vi "UHR-Fleezers Control (fpga) - Leonardo 04-2018 V4b_AlexFCS.vi"() -> ()   [LabVIEW 2013]
doc: "UHR-Fleezers Instrument Control Code (fpga)"
uses:
  <vilib>/Platform/TimedLoop/XDataNode/timing_clust.ctl
  <vilib>/Platform/TimedLoop/XDataNode/nitl_modes.ctl
  <vilib>/Platform/TimedLoop/XDataNode/wakeup.ctl
  <vilib>/rvi/eio/common/nirviEmuTemplateMethod_errors.vi
  <vilib>/rvi/Emulation/niFpgaSctlEmulationGetInTimedLoop.vi
  <vilib>/rvi/Emulation/niFpgaEmulationReportErrorSimple.vi
  <vilib>/rvi/Emulation/niFpgaGetClockAttributes.vi
  <vilib>/rvi/Emulation/niFpgaCriticalErrorInLSC.vi
  <vilib>/rvi/FIFO/Fifo_Resource/nirvififoEmulationReadFpgaImpl.vi
  <vilib>/rvi/DataTransferAndStorage/Container/Common/niFpgaContainerGetUniqueNameForEmu.vi
  <vilib>/rvi/DataTransferAndStorage/Container/Common/niFpgaContainerExecOnDevCompGetState.vi
  <vilib>/rvi/interface/RandomDataEmulation/nirviRandomDataFPGAFIFO.vi
  <vilib>/rvi/interface/RandomDataEmulation/niFpgaRandomDataHandleErrors.vi
  <vilib>/rvi/eio/common/nirviEmuReportErrorAndStop.vi
  <vilib>/rvi/FIFO/Fifo_Resource/nirvififoEmulationGetNumberOfElementsToReadFpgaImpl.vi
  <vilib>/rvi/FIFO/Fifo_Resource/nirvififoEmulationClearFpgaImpl.vi
  <vilib>/rvi/Emulation/niFpgaProcessEmulError.vi
  <vilib>/rvi/FIFO/Fifo_Resource/nirvififoEmulationWriteFpgaImpl.vi
  <vilib>/Platform/TimedLoop/XDataNode/XDataNode.xnode
  <vilib>/eio/EIOMethodNode/EIOMethodNode.xnode
  <vilib>/eio/EIONode/EIONode.xnode
  <vilib>/rvi/DataTransferAndStorage/Container/XNode/niFpgaContainer.xnode
  <vilib>/rvi/FIFO/Fifo_Resource/nirvififoEmulationRead.vi
  <vilib>/rvi/FIFO/Fifo_Resource/niFpgaFifoEmulationRefIn.vi
  <vilib>/rvi/FIFO/Fifo_Resource/nirvififoEmulationGetNumberOfElementsToRead.vi
  <vilib>/rvi/interface/RandomDataEmulation/nirviRandomDataFpgaReadWriteTemplate.vi
  <vilib>/rvi/FIFO/Fifo_Resource/nirvififoEmulationWrite.vi
  <vilib>/addons/control/pid/fpga.llb/XNode/niFpgaPID.xnode
  <vilib>/Platform/TimedLoop/XDataNode/XDNodeRunTimeDep.lvlib
  <vilib>/rvi/Memory/Memory_Emulation/niFpgaMemoryEmulationRefIn.vi
panel:
  in  "Tab Control 2":T1(tab)
  out "BD1 amplitude 1 out":u16
  out "BD1 amplitude 2 out":u16
  in  "FB output range":cluster{"output low":i16, "output high":i16}={"output low"=0, "output high"=3000}
  in  "FB Gains":T2={"proportional gain (Kc)"=10, "integral gain (Kc*Ts/Ti)"=5, "derivative gain (Kc*Td/Ts)"=0}
  in  "RF synth green feedback max":i16=4000
  in  "RD":bool=TRUE
  in  "Swap F1 and F2":bool
  in  "Scan BD":bool
  in  "Start scan":bool
  in  "OSK Bd 1":bool
  in  "Reset Bd 1":bool
  in  "PMODE":bool=TRUE
  in  "Number Interlace Cycles":u8=2 min=1 max=3
  in  "Interlace Off Parameters":u8=1 min=1 max=3
  in  "Interlace ON/OFF":bool
  out "DIO Relative phase":i16
  in  "Phase count adjustment (DIO)":i16
  in  "+ phase (DIO)":bool
  out "DIO Late Counter":u8
  in  "DIO count 1 (ticks)":u16=400
  in  "DIO count 2 (ticks)":u16=400
  in  "DIO count 3 (ticks)":u16=400
  out "AI2 Y Sum Set 2":i16
  out "AI2 Y Sum Set 1":i16
  in  "FB Setpoint Set 1":i16 min=0 step=1
  in  "FB Reset Set 1":bool
  in  "FB On/Off Set 1":bool
  in  "FB Reset Set 2":bool
  in  "FB On/Off Set 2":bool
  in  "FB Setpoint Set 2":i16 min=0 step=1
  in  "Amp switch delay":u8=5
  in  "RF synth bd controls green":bool
  in  "Phase Trap 2":fxp<+,14,14>
  in  "Phase Trap 1":fxp<+,14,14>
  in  "Phase offset method":u8
  in  "BD 2 Amplitude 1":u16
  in  "BD 1 Amplitude 1":u16
  in  "BD 2 Frequency 1":u64
  in  "BD 1 Frequency 1":u64
  in  "BD 2 Amplitude 2":u16
  in  "BD 1 Amplitude 2":u16
  in  "BD 2 Frequency 2":u64
  in  "BD 1 Frequency 2":u64
  in  "BD 2 Amplitude 3":u16
  in  "BD 1 Amplitude 3":u16
  in  "BD 2 Frequency 3":u64
  in  "BD 1 Frequency 3":u64
  in  "BD 2 Delay (Ticks)":u8 caption="Count(Ticks)"
  in  "Next trap write delay (ticks)":u8 caption="Count(Ticks)"
  out "Random phase generated":fxp<+,14,14>
  in  "RF phase reset before cycles":bool
  in  "Trap 1 osc enable":bool
  in  "N trap osc periods":i16
  in  "Trap osc period (pts)":i16
  in  "Osc traps":bool
  in  "Initiate trap osc":bool
  in  "Ready Write":bool
  in  "Data":i64
  in  "Address 2":u32
  in  "Osc trap cont.":bool
  in  "Trap 2 osc enable":bool
  out "green FB running":bool
  in  "APD 2 AO scale factor":i16=1
  in  "BD 1 Delay (ticks)":u8
  in  "Tab Control":T3(tab)=enum."MCL trap control"
  in  "Set 3":bool
  in  "Set 2":bool=TRUE
  in  "Set 1":bool=TRUE
  in  "Trap Pos to FIFO":bool
  in  "N of AI1 Int Acq Sets":i16=2 min=1 max=3 step=1
  out "AI Late Counter":u8
  in  "ai count":u16=400
  in  "+ phase":bool
  in  "Phase count adjustment":i16
  out "Relative phase":i16
  in  "AI to FIFO":bool
  out "BD1 Frequency Out 1":u64
  out "BD1 Frequency Out 2":u64
  out "Trap Pos FIFO Timeout":u16
  out "Trap AI FIFO Timeout":u16
  in  "Trap FIFO Set Timeout":i32
  in  "Scan freq.  increment":i64
  in  "Scan steps":u64
  in  "Number of scans":u16
  in  "Cycles per step":u64
  in  "Raster setpoint":fxp<+/-,16,1>
  in  "Raster to target force":bool
  out "Actual Scan freq":u64
  in  "Cont. Scan":bool
  out "Scan I":u64
  in  "Abort scan":bool
  out "Scanning":bool
  in  "FB Min frequency":u64
  in  "FB Max Frequency":u64
  in  "Dynamic Force FB (Ronen)":bool
  in  "Trap pos. FB Range":T4={"FB2 output low"=-1.0, "FB2 output high"=0.999969482421875}
  in  "Trap Pos. FB Gains":T5={"proportional gain (Kc)"=0.999969482421875, "integral gain (Kc*Ts/Ti)"=0.999969482421875, "derivative gain (Kc*Td/Ts)"=0.0}
  in  "B factor":fxp<+/-,32,16>
  in  "Negate Diff?":bool
  in  "Diff FB Measurement?":bool
  in  "FB Trig Integrate":u32=1
  out "TTrig?":bool
  in  "TTrig Negate Pos":bool=TRUE
  out "Trap Pos FB Int Signal":fxp<+/-,24,9> format="%.18g"
  out "Trap Pos FB Int-Norm Signal":fxp<+/-,16,1> format="%.16g"
  in  "FPGA TTrig Thresh":i64
  in  "FPGA Trap Trig":bool
  out "Trap Pos FB Action":i64
  in  "Trap Pos. FB Offset Factor":i64
  in  "Trap Pos. FB Mult Factor":i64=2
  in  "Trap Pos. FB Reset":bool
  in  "Trap Pos FB Monitor T1 or T2":bool
  in  "AI1 X Scale":u16
  in  "Trap Pos FB Int Count":u16=100
  in  "Trap Pos FB Negate Action":bool
  out "AI1 X Set 2":fxp<+/-,16,1>
  out "AI1 X Set 1":fxp<+/-,16,1>
  in  "Trap Pos. FB SP":fxp<+/-,16,1>
  in  "Force feedback":bool
  out "TTrig Sig":i64
  out "TTrig Fin Thresh":i64
  in  "1D or 2D Scan?":bool
  in  "Abort scan (MCL)":bool
  in  "MCL Scan Axis":bool
  in  "Cont. Scan (MCL)":bool
  out "Scan I (MCL)":u64
  in  "Number of scans (MCL)":u16
  out "Scanning MCL":bool
  in  "Scan steps (MCL)":u64
  in  "Cycles per step (MCL)":u64
  in  "Scan freq.  increment (MCL)":i16
  in  "Start scan (MCL)":bool
  in  "AO2 (X)":i16
  in  "AO1 (Y)":i16
  out "MCL Late Counter":u8
  in  "MCL count":u32=800
  out "MCL Relative Phase":i16
  in  "Phase count adjustment (MCL)":i16
  in  "+ phase (MCL)":bool
  in  "Lifetime events to read blue":u16=100
  in  "Lifetime read blue fifo":bool
  out "lifetime events in fifo":u16
  out "APD2 int gate":bool
  in  "APD Gate Operating Mode":u8 max=2 step=1
  in  "Invert APD Gate":bool
  in  "APD Gate OFF Count":u16=100
  in  "APD Gate ON Count":u16=300
  out "APD 1 Gate Late Counter":u8
  out "APD 1 Gate Relative Phase":i16
  in  "Phase count adjustment (APD 1 Gate)":i16
  in  "+ phase (APD 1 Gate)":bool
  in  "Phase count adjustment (APD 2 Gate)":i16
  out "APD 2 Gate Late Counter":u8
  out "APD 2 Gate Relative Phase":i16
  in  "+ phase (APD 2 Gate)":bool
  out "APD 3 Counts 0":u32
  out "APD 3 Counts 1":u32
  out "APD 3 Gate Late Counter":u8
  in  "Phase count adjustment (APD 3 Gate)":i16
  out "APD 3 Gate Relative Phase":i16
  in  "+ phase (APD 3 Gate)":bool
  out "APD1 int gate":bool
  out "APD3 int gate":bool
  in  "Lifetime timeout APD1":u16=200
  in  "APD to FIFO":bool
  in  "APD Acq Rate Count":u32=20000000
  out "APD Acq Late Counter":u16
  out "APD Acq Relative Phase":i16
  in  "+ phase (APD Acq)":bool
  in  "Phase Count Adjustment (APD Acq)":i16
  in  "APD 1 AO scale factor":i16=1
  out "APD Acq Late?":bool
  in  "Number of OFF cycles":i16
  in  "Green long-scale interlacing":bool
  in  "D3 2":i16
  in  "I3 2":i16=5
  in  "P3 2":i16=10
  in  "Green FB Setpoint 2":i16=250 min=0 step=1
  in  "Green FB Reset 2":bool
  in  "Green Filter Flipper":bool
  in  "Green interlace OFF count":u16=100
  out "GI Relative phase":i16
  in  "Phase count adjustment (GI)":i16
  in  "+ phase (GI)":bool
  in  "Green interlace ON count":u16=300
  out "GI Late Counter":u8
  in  "Invert GI":bool
  in  "Operating Mode":u8 max=2 step=1
  in  "Current Out":u16=30000
  in  "Green int current ON count adj":u32=150
  in  "Green interlace OFF count 2":u32=900
  in  "Green interlace ON count 2":u32=300
  out "GI Late Counter 2":u16
  in  "Green FB Count":u32=1200
  in  "Phase count adjustment (GI) 2":i16=20
  in  "Green FB Setpoint":i16=250 min=0 step=1
  in  "Invert GI 2":bool
  out "GI Relative phase 2":i16
  in  "+ phase (GI) 2":bool
  in  "Phase count adjustment (Green FB)":i16=10
  out "Green Late Counter":u16
  out "Green FB Relative Phase":i16
  in  "+ phase (Green FB)":bool
  out "Green FB Signals":T6
  out "Green FB Sum":i16
  in  "Green FB Gains":T2={"proportional gain (Kc)"=10, "integral gain (Kc*Ts/Ti)"=5, "derivative gain (Kc*Td/Ts)"=0}
  in  "Green FB On/Off":bool
  in  "Green FB Reset":bool
  out "Green FB Late?":bool
  out "GI Late?":bool
  in  "Operating Mode 2":u8=2 max=2 step=1
  in  "Chassis2/Mod4/AO1":u16
  in  "Number of ON cycles":i16
  in  "+ phase (RI)":bool
  out "RI Relative phase":i16
  out "RI Late Counter":u8
  in  "Red interlace ON count":u16=300
  in  "Red interlace OFF count":u16=100
  in  "Invert RI":bool
  in  "Red Laser Operating Mode":u8 max=2 step=1
  in  "Phase count adjustment (RI)":i16
  in  "Phase count adjustment (BI D)":i16
  in  "Blue Laser Operating Mode (D)":u8 max=2 step=1
  in  "Invert BI (D)":bool
  in  "Blue interlace OFF count (D)":u16=100
  in  "Blue interlace ON count (D)":u16=300
  out "Blue Late Counter (D)":u8
  out "BI Relative phase (D)":i16
  in  "+ phase (BI D)":bool
  in  "Lifetime to FIFO":bool
  out "lifetime (ticks)":u16
  # "Raster Scan AOD"
  # "1 (X)"
  # "2 (Y)"
  # "IR Intensity Feedback (RF BD 1)"
  # "FB Gains Set 1"
  # "FB output range 1"
  # "IR Intensity Feedback (RF BD 2) -\nonly when using BD 2 for green laser AOM (not trap Y)"
  # "Keep below 4096 (12 bits) to stay within range of RF board. Going over doesn't saturate, it truncates higher bits."
  # "RF phase offset control"
  # "Methods are:\n0 - Default, do nothing at all (no phase offset writes)\n1 - Manual phase adjustment\n2 - Cycle the phase adjustment using the input phase numbers as increment values for each cycle"
  # "False is usual, True is external loop method"
  # "Parameters if using the external RF switching loop"
  # "Parameters if using the usual internal RF switching method"
  # "FB Triggering Excitation Laser"
  # "Trap Pos. FB Gains"
  # "Trap Pos. FB Range"
  # "AO1 (Y)"
  # "2D"
  # "Trap 3"
  # "1D"
  # "AO2 (X)"
  # "Fl Laser"
  # "APD AO for aligning"
  # "Detection Loop"
  # "Green fluorescent laser digital gate interlacing loop"
  # "0 Forced ON\n1 Forced OFF\n2 Interlacing"
  # "ALEX settings:"
  # "Controls for usual IA ME controls green AOM"
  # "Controls for RF synth board controls green AOM"
  # "Green FB Gains"
  # "Red fluorescent laser digital gate interlacing loop"
  # "Detection Loop"
  # "0 Forced ON\n1 Forced OFF\n2 Interlacing"
  # "Analog/FB Control Loop\n(Disabled)"
  # "Digital Control Loop"
  # "Blue laser intensity reading"
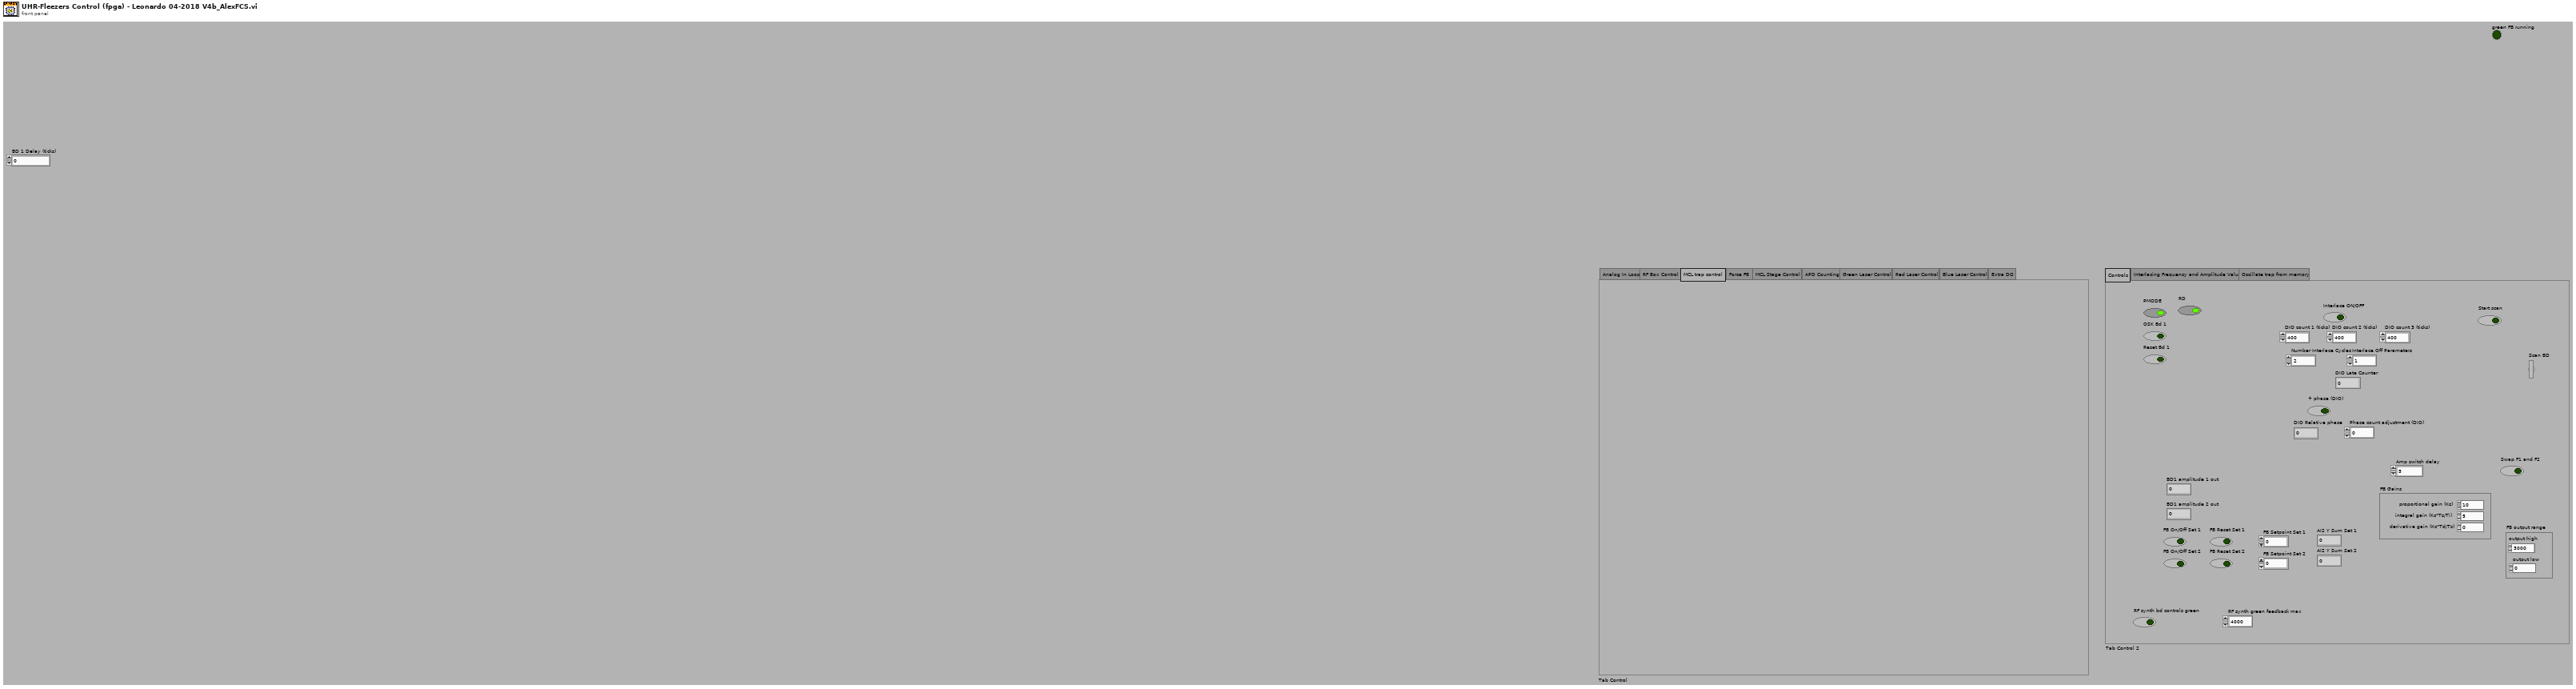
[diagram p1: front panel]
types:
  T1 = enum32{"Controls", "Interlacing Frequency and Amplitude Values", "Oscillate trap from memory"}
  T2 = cluster{"proportional gain (Kc)":i16, "integral gain (Kc*Ts/Ti)":i16, "derivative gain (Kc*Td/Ts)":i16}
  T3 = enum32{"Analog In Loop", "RF Box Control", "MCL trap control", "Force FB", "MCL Stage Control", "APD Counting", "Green Laser Control", "Red Laser Control", "Blue Laser Control", "Extra DO"}
  T4 = cluster{"FB2 output low":fxp<+/-,16,1>, "FB2 output high":fxp<+/-,16,1>}
  T5 = cluster{"proportional gain (Kc)":fxp<+/-,16,1>, "integral gain (Kc*Ts/Ti)":fxp<+/-,16,1>, "derivative gain (Kc*Td/Ts)":fxp<+/-,16,1>}
  T6 = cluster{"Green FB Ch 0":i16, "Green FB Ch 1":i16, "Green FB Ch 2":i16}
  T7 = typedef "XDNodeRunTimeDep.lvlib/timing_clust.ctl" = cluster{"Expected End [f-1]":u64, "Actual End [f-1]":u64, "Finished Late? [f-1]":bool, "Expected End [i-1]":u64, "Actual End [i-1]":u64, "Finished Late? [i-1]":bool, "Expected Start [i]":u64, "Actual Start [i]":u64, "Expected Start [f]":u64, "Actual Start [f]":u64, "Source Name":string, "Structure Name":string, "Period":i64, "Deadline":i64, "Offset":i64, "Start":i64, "Priority":i32, "Timeout":i32, "Mode":T8, "Wakeup Reason":T9, "Error":errorcluster, "Source Type":string, "Secondary Source Type":string, "Global End Time":u64, "Global Start Time":u64, "Frame Duration":u64, "Iteration Duration":u64, "Assigned CPU":i32, "I/O Scan Engine Mode":u32}
  T8 = typedef "XDNodeRunTimeDep.lvlib/nitl_modes.ctl" = enum32{"No Change", "Process missed periods, maintain original phase", "Discard missed periods, maintain original phase", "Process missed periods, ignore original phase", "Discard missed periods, ignore original phase"}
  T9 = typedef "XDNodeRunTimeDep.lvlib/wakeup.ctl" = enum32{"Normal", "Aborted", "Asynchronous wakeup", "Timing source error", "Timed loop error", "Timeout"}
  T10 = cluster{"Chassis2/Mod2/AI0":i16, "Chassis2/Mod2/AI1":i16, "Chassis2/Mod2/AI2":i16}
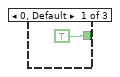
[diagram p4: hidden frame]
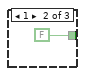
[diagram p5: hidden frame]
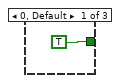
[diagram p8: hidden frame]
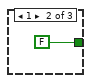
[diagram p9: hidden frame]
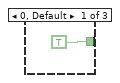
[diagram p13: hidden frame]
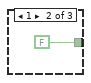
[diagram p14: hidden frame]
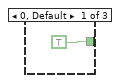
[diagram p15: hidden frame]
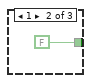
[diagram p16: hidden frame]
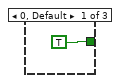
[diagram p20: hidden frame]
diagram:
  w7 = FALSE
  w8 = FALSE
  # "BD2 amp"
  # "BD1 amp"
  # "BD2 amp"
  # "BD1 amp"
  # "timing array current index"
  # "timing array"
  # "timing counter (phase adjusted here)"
  # "late counter"
  n1 = while {
    stop <- FALSE stop-if-true
    n2 = xnode "FPGA I/O Node"("Connector0/DIO3"="Green Filter Flipper", "Chassis2/Mod1/AO1"="Chassis2/Mod4/AO1") -> ()  [unwired: 2 in, 2 out]
    n3 = call "Loop Timer11"("Count(Ticks)"=u32 40000 ("Extra DO Counts")) -> ()  [unwired: 1 out]
  }
  n4 = disable-structure shown="Disabled" {
    frame Disabled {
      w22 = i16 2 items=["UnSet Ready", "ReadWrite", "Wait Ready"]
      n5 = while "Handshake memory transfer for trap oscillation sin wave data" {
        shift-right: [w24] -> _
        shift-left: w22 -> [w25]
        stop <- FALSE stop-if-true
        # "Write"
        n6 = case shown="1" w25 {
          tunnel: [w28 w33 w34] -> w24
          frame 3, Default {
            w26 = i16 2 items=["UnSet Ready", "ReadWrite", "Wait Ready"]
            w27 = i16 1 items=["UnSet Ready", "ReadWrite", "Wait Ready"]
            n7 = Select(t=w27, s="Ready Write", f=w26) -> (s? t:f=w28:i16)
          }
          frame 1 {
            w33 = i16 0 items=["UnSet Ready", "ReadWrite", "Wait Ready"]
            n8 = xnode ("Memory Write")("Address"="Address 2", "Data"="Data", "Memory In"=refnum<k21> "Trap osc memory") -> ()  [unwired: 1 out]
          }
          frame 0 {
            w34 = i16 2 items=["UnSet Ready", "ReadWrite", "Wait Ready"]
            n9 = local write "Ready Write"(FALSE ("Ready Read")) -> ()
          }
        }
      }
    }
    frame Enabled {
    }
  }
  n10 = flat-sequence "FPGA initialization to do before running any of the loops" {
    tunnel: [u16 0 ("DIO count 3 (ticks)")] -> w6
    tunnel: [w43] -> _
    frame #0 {
      # "UDCLK out enable and set low"
      # "WR"
      # "BD 2"
      # "BD 1"
      # "With the RF synth board initialization now done in a separate fpga vi, now when this vi is started, board is already configured and is ready for interlacing. Just need to set WR high and enabled UDCLK as write and set to low.\nbefore setting data and address bits."
      # "Start up expansion chassis early\nto avoid delays later"
      # "Set data and address values to something safe (a correct setting) so any initial WR and udclk flipping doesn't have a chance to mess anything up. Safe would be setting an unused data entry:"
      n11 = xnode "FPGA I/O Method Node"("Enable"=TRUE) -> ("FPGA I/O Out"=w37:refnum<k21>)  [unwired: 1 in]
      n12 = xnode "FPGA I/O Method Node"("Enable"=TRUE) -> ("FPGA I/O Out"=w40:refnum<k21>)  [unwired: 1 in]
      n13 = xnode "FPGA I/O Node"("Chassis2/Mod1/AO0"=u16 0 ("Chassis2/Mod4/AO0")) -> ("Chassis2/Mod2/AI0"=w43:i16)  [unwired: 2 in, 2 out]
      n14 = xnode "FPGA I/O Node"("Connector1/DIO15"=TRUE) -> ()  [unwired: 1 in, 1 out]
      n15 = xnode "FPGA I/O Node"("I/O Item"=FALSE ("Connector1/DIO30"), "FPGA I/O In"=w37) -> ()  [unwired: 1 out]
      n16 = xnode "FPGA I/O Node"("I/O Item"=FALSE ("Connector1/DIO30"), "FPGA I/O In"=w40) -> ()  [unwired: 1 out]
      n17 = xnode "FPGA I/O Node"("Connector1/DIO0"=FALSE, "Connector1/DIO1"=FALSE, "Connector1/DIO2"=FALSE, "Connector1/DIO3"=FALSE, "Connector1/DIO4"=FALSE, "Connector1/DIO5"=FALSE, "Connector1/DIO6"=FALSE, "Connector1/DIO7"=FALSE, "Connector1/DIO8"=FALSE, "Connector1/DIO9"=FALSE, "Connector1/DIO10"=FALSE, "Connector1/DIO11"=FALSE, "Connector1/DIO12"=FALSE, "Connector1/DIO13"=FALSE, "Connector1/DIO20"=FALSE, "Connector1/DIO21"=FALSE, "Connector1/DIO22"=FALSE, "Connector1/DIO23"=FALSE, "Connector1/DIO24"=FALSE, "Connector1/DIO25"=FALSE, "Connector1/DIO26"=FALSE, "Connector1/DIO27"=FALSE, "Connector1/DIO14"=FALSE) -> ()  [unwired: 23 in, 23 out]
    }
  }
  n18 = node-c288() -> (w14:T7)  [unwired: 1 in]
  n19 = timed-loop "RF box board DIO control: control bits" {
    timing: w14 -> [_]
    timing-out: [_] -> w13
    tunnel: [w70] -> _
    tunnel: w6 -> [w70]
    stop <- FALSE stop-if-true
    n20 = xnode "FPGA I/O Node"("Connector1/DIO16"="RD", "Connector1/DIO17"="PMODE", "Connector1/DIO18"="OSK Bd 1", "Connector1/DIO19"="Reset Bd 1") -> ()  [unwired: 4 in, 4 out]
  }
  n21 = node-c288(w13) -> ()
  n22 = local read "AO1 (Y)"() -> (w16:i16)
  n23 = local read "AO2 (X)"() -> (w15:i16)
  n24 = node-c288() -> (w2:T7)  [unwired: 1 in]
  n25 = node-c288() -> (w4:T7)  [unwired: 1 in]
  n26 = To Unsigned Long Integer(number=w6) -> (unsigned 32bit integer=w9:u32)
  n27 = disable-structure shown="Disabled" {
    disable-tunnel: w8 -> [w78 _]
    disable-tunnel: w6 -> [w77 _]
    frame Disabled {
      n28 = while "APD 2 Gating" {
        shift-right: [w82] -> _
        shift-left: w77 -> [w87]
        shift-right: [w81] -> _
        shift-left: w78 -> [w79]
        stop <- FALSE stop-if-true
        n29 = flat-sequence {
          tunnel: w87 -> [w90]
          tunnel: [w91] -> w85
          tunnel: [w90] -> w83
          tunnel: [w89] -> w80
          tunnel: w79 -> [w89]
          tunnel: [w94] -> w86
          tunnel: w85 -> [w94]
          tunnel: [w93] -> w84
          tunnel: w83 -> [w93]
          tunnel: w80 -> [w92]
          tunnel: [w116] -> w82
          tunnel: w86 -> [w126]
          tunnel: w84 -> [w124]
          tunnel: [w95] -> w81
          frame #0 {
            n30 = call "Loop Timer3"("Count(Ticks)"=w90) -> ("Tick Count(Ticks)"=w91:u32)
          }
          frame #1 {
            # "Signal maybe then sent through \na transistor before APD"
            n31 = xnode "FPGA I/O Node"("Connector1/DIO34"=w92) -> ()  [unwired: 1 in, 1 out]
            "APD2 int gate" <- w92
          }
          frame #2 {
            n32 = local read "APD Gate ON Count"() -> (w109:u16)
            n33 = local read "APD Gate OFF Count"() -> (w108:u16)
            n34 = feedback #1(TRUE) -> (w121:bool)
            n35 = feedback-in #2(w126) -> ()
            n36 = feedback #2(w126) -> (w110:u32)
            n37 = Not(x=w121) -> (.not. x?=w119:bool)
            n38 = feedback-in #1(w119) -> ()
            n39 = Subtract(x=w126, y=w110) -> (x-y=w125:u32)
            n40 = Select(t=w109, s=w119, f=w108) -> (s? t:f=w123:u16)
            n41 = Subtract(x=w125, y=w124) -> (x-y=w101:u32)
            n42 = Subtract(x=w123, y=w101) -> (x-y=w115:u32)
            n43 = Number To Boolean Array(number=w101) -> (Boolean array=w100:bool[])
            n44 = Or Array Elements(Boolean array=w100) -> (logical OR=w99:bool)
            n45 = Boolean To (0,1)(Boolean="+ phase (APD 2 Gate)") -> (0, 1=w113:i16)
            n46 = Multiply(x=w113, y="Phase count adjustment (APD 2 Gate)") -> (x*y=w111:i16)
            n47 = Boolean To (0,1)(Boolean=w99) -> (0, 1=w106:i16)
            n48 = Add(x=w115, y=w111) -> (x+y=w116:u32)
            n49 = To Unsigned Byte Integer(number=w106) -> (unsigned 8bit integer=w103:u8)
            n50 = feedback #3(i16 0) -> (w118:i16)
            n51 = Subtract(x=w118, y=w111) -> (x-y=w117:i16)
            "APD 2 Gate Relative Phase" <- w117
            n52 = feedback-in #3(w117) -> ()
            n53 = feedback #4(u8 0) -> (w104:u8)
            n54 = Add(x=w103, y=w104) -> (x+y=w102:u8)
            "APD 2 Gate Late Counter" <- w102
            n55 = feedback-in #4(w102) -> ()
            n56 = local read "APD Gate Operating Mode"() -> (w107:u8)
            n57 = case shown="2" w107 {
              tunnel: [TRUE FALSE w129] -> w96
              tunnel: w121 -> [_ _ w129]
              frame 0, Default {
              }
              frame 1 {
              }
              frame 2 {
              }
            }
            n58 = local read "Invert APD Gate"() -> (w98:bool)
            n59 = Not(x=w96) -> (.not. x?=w97:bool)
            n60 = Select(t=w97, s=w98, f=w96) -> (s? t:f=w95:bool)
          }
        }
      }
    }
    frame Enabled {
    }
  }
  n61 = while "DAQ AI set 1" {
    shift-right: [w130] -> _
    shift-left: w6 -> [w135]
    stop <- FALSE stop-if-true
    n62 = flat-sequence {
      tunnel: w135 -> [w146]
      tunnel: [w145] -> w133
      tunnel: [w146] -> w132
      tunnel: [w156] -> w143
      tunnel: [w155] -> w142
      tunnel: [w154] -> w141
      tunnel: [w153] -> w140
      tunnel: [w152] -> w139
      tunnel: [w151] -> w138
      tunnel: [w150] -> w137
      tunnel: [w149] -> w136
      tunnel: [w148] -> w134
      tunnel: w133 -> [w148]
      tunnel: w132 -> [w147]
      tunnel: [w147] -> w131
      tunnel: [w186] -> w130
      tunnel: w143 -> [w212]
      tunnel: w142 -> [w178]
      tunnel: w141 -> [w179]
      tunnel: w140 -> [w158]
      tunnel: w139 -> [w202]
      tunnel: w138 -> [w201]
      tunnel: w137 -> [w200]
      tunnel: w136 -> [w199]
      tunnel: w134 -> [w196]
      tunnel: w131 -> [w193]
      frame #0 {
        n63 = call "Loop Timer"("Count(Ticks)"=w146) -> ("Tick Count(Ticks)"=w145:u32)
      }
      frame #1 {
        n64 = xnode "FPGA I/O Node"("Connector1/DIO31"=TRUE ("Connector1/DIO33")) -> ("Connector0/AI0"=w156:i16, "Connector0/AI1"=w155:i16, "Connector0/AI2"=w154:i16, "Connector0/AI3"=w153:i16, "Connector0/AI4"=w152:i16, "Connector0/AI5"=w151:i16, "Connector0/AI6"=w150:i16, "Connector0/AI7"=w149:i16)  [unwired: 9 in, 9 out]
      }
      frame #2 {
        w182 = FALSE ("AI to FIFO")
        # "Normalize by trap bead QPD sum, AI3"
        # "Adjust phase after data acquired if button pressed"
        n65 = feedback #5(i16 1) -> (w205:i16)
        n66 = Increment(x=w205) -> (x+1=w211:i16)
        n67 = Scale By Power Of 2(n="AI1 X Scale", x=w178) -> (x*2^n=w176:i16)
        n68 = Greater?(x=w211, y="N of AI1 Int Acq Sets") -> (0:w208:bool)
        n69 = Select(t=i16 1, s=w208, f=w211) -> (s? t:f=w210:i16)
        n70 = feedback-in #5(w210) -> ()
        n71 = Divide(x=w176, y=w158) -> (x/y=w175:fxp<+/-,16,1>)
        n72 = feedback #6(w182) -> (w180:bool)
        n73 = feedback #7(w182) -> (w198:bool)
        n74 = case shown="1, Default" w205 {
          tunnel: w179 -> [w235 w242 _]
          tunnel: ["Set 1" "Set 2" "Set 3"] -> w203
          tunnel: ["AI to FIFO" w244 w249] -> w197
          tunnel: w198 -> [_ w244 w249]
          tunnel: ["Trap Pos to FIFO" w243 w248] -> w181
          tunnel: w180 -> [_ w243 w248]
          tunnel: w175 -> [w234 w241 _]
          tunnel: [w233 w239 FALSE] -> w162
          tunnel: [w232 w240 u64 0 ("BD1 Frequency Out 2")] -> w161
          frame 1, Default {
            n75 = local read "BD1 Frequency Out 1"() -> (w232:u64)
            n76 = Compound Arithmetic op=AND("Trap Pos to FIFO", "Set 1", "AI to FIFO") -> (w233:bool)
            "AI2 Y Sum Set 1" <- w235
            "AI1 X Set 1" <- w234
          }
          frame 2 {
            n77 = local read "BD1 Frequency Out 2"() -> (w240:u64)
            n78 = Compound Arithmetic op=AND(w243, "Set 2", w244) -> (w239:bool)
            "AI2 Y Sum Set 2" <- w242
            "AI1 X Set 2" <- w241
          }
          frame 3 {
          }
        }
        n79 = And(x=w203, y=w197) -> (x .and. y?=w204:bool)
        n80 = case shown="True" w204 {
          tunnel: w212 -> [_ w263]
          tunnel: w178 -> [_ w262]
          tunnel: w179 -> [_ w261]
          tunnel: w158 -> [_ w260]
          tunnel: w202 -> [_ w259]
          tunnel: w201 -> [_ w258]
          tunnel: w200 -> [_ w257]
          tunnel: w199 -> [_ w256]
          tunnel: 0 ("DMA buffer timeout") -> [_ w265]
          frame False {
          }
          frame True {
            n81 = Build Array(w263, w262, w261, w260, w259, w258, w257, w256) -> (w264:i16[])
            n82 = for {
              tunnel: w264 -> [w267] mode=indexing
              tunnel: w265 -> [w268]
              tunnel: [w266] -> w254 mode=indexing
              n83 = xnode ("FIFO Write")("Element"=w267, "Timeout"=w268) -> ("Timed Out?"=w266:bool)  [unwired: 1 in, 1 out]
            }
            n84 = Or Array Elements(Boolean array=w254) -> (logical OR=w251:bool)
            n85 = Boolean To (0,1)(Boolean=w251) -> (0, 1=w253:i16)
            n86 = feedback #8(u16 0) -> (w252:u16)
            n87 = Add(x=w253, y=w252) -> (x+y=w250:u16)
            "Trap AI FIFO Timeout" <- w250
            n88 = feedback-in #8(w250) -> ()
          }
        }
        n89 = feedback-in #6(w181) -> ()
        n90 = feedback-in #7(w197) -> ()
        n91 = case shown="True" w162 {
          tunnel: w161 -> [_ w218]
          tunnel: [u8 0 w215] -> w160
          frame False {
          }
          frame True {
            n92 = Split Number(x=w218) -> (hi(x)=w219:u32, lo(x)=w220:u32)
            n93 = Split Number(x=w219) -> (lo(x)=w221:u16)  [unwired: 1 out]
            n94 = Split Number(x=w220) -> (hi(x)=w222:u16, lo(x)=w223:u16)
            n95 = Build Array "BD 1 nu Stack"(w221, w222, w223) -> (w217:u16[])
            n96 = for {
              tunnel: w217 -> [w230] mode=indexing
              shift-right: [w226] -> w215
              shift-left: u8 0 -> [w227]
              n97 = xnode ("FIFO Method Node")("Element"=w230, "Timeout"="Trap FIFO Set Timeout") -> ("Timed Out?"=w229:bool)  [unwired: 1 in, 1 out]
              n98 = Boolean To (0,1)(Boolean=w229) -> (0, 1=w228:i16)
              n99 = To Unsigned Byte Integer(number=w228) -> (unsigned 8bit integer=w225:u8)
              n100 = Add(x=w225, y=w227) -> (x+y=w226:u8)
            }
          }
        }
        n101 = To Unsigned Word Integer(number=w160) -> (unsigned 16bit integer=w159:u16)
        n102 = feedback #9(u16 0) -> (w173:u16)
        n103 = Add(x=w159, y=w173) -> (x+y=w172:u16)
        "Trap Pos FIFO Timeout" <- w172
        n104 = feedback-in #9(w172) -> ()
        n105 = feedback-in #10(w196) -> ()
        n106 = feedback #10(w196) -> (w195:u32)
        n107 = Subtract(x=w196, y=w195) -> (x-y=w194:u32)
        n108 = xnode "FPGA I/O Node"("Connector1/DIO31"=FALSE ("Connector1/DIO34")) -> ()  [unwired: 1 in, 1 out]
        n109 = Subtract(x=w194, y=w193) -> (x-y=w164:u32)
        n110 = Boolean To (0,1)(Boolean="+ phase") -> (0, 1=w189:i16)
        n111 = Multiply(x=w189, y="Phase count adjustment") -> (x*y=w183:i16)
        n112 = Subtract(x="ai count", y=w164) -> (x-y=w187:u32)
        n113 = Number To Boolean Array(number=w164) -> (Boolean array=w165:bool[])
        n114 = feedback #11(i16 0) -> (w185:i16)
        n115 = Add(x=w187, y=w183) -> (x+y=w186:u32)
        n116 = Subtract(x=w185, y=w183) -> (x-y=w184:i16)
        "Relative phase" <- w184
        n117 = feedback-in #11(w184) -> ()
        n118 = Or Array Elements(Boolean array=w165) -> (logical OR=w163:bool)
        n119 = Boolean To (0,1)(Boolean=w163) -> (0, 1=w170:i16)
        n120 = To Unsigned Byte Integer(number=w170) -> (unsigned 8bit integer=w167:u8)
        n121 = feedback #12(u8 0) -> (w168:u8)
        n122 = Add(x=w167, y=w168) -> (x+y=w166:u8)
        "AI Late Counter" <- w166
        n123 = feedback-in #12(w166) -> ()
      }
    }
  }
  n124 = while "MCL stage control" {
    shift-right: [w281] -> _
    shift-left: w6 -> [w284]
    shift-right: [w274] -> _
    shift-left: w16 -> [w271]
    shift-right: [w273] -> _
    shift-left: w15 -> [w269]
    stop <- FALSE stop-if-true
    n125 = flat-sequence {
      tunnel: w284 -> [w287]
      tunnel: [w286] -> w280
      tunnel: [w287] -> w278
      tunnel: [w289] -> w272
      tunnel: w271 -> [w289]
      tunnel: [w288] -> w270
      tunnel: w269 -> [w288]
      tunnel: w280 -> [w293]
      tunnel: [w293] -> w279
      tunnel: w278 -> [w292]
      tunnel: [w292] -> w277
      tunnel: w272 -> [w291]
      tunnel: w270 -> [w290]
      tunnel: w279 -> [w301]
      tunnel: w277 -> [w300]
      tunnel: [w301] -> w283
      tunnel: [w300] -> w282
      tunnel: [w299] -> w276
      tunnel: [w298] -> w275
      tunnel: [w373] -> w281
      tunnel: w283 -> [w380]
      tunnel: w282 -> [w377]
      tunnel: w276 -> [w375]
      tunnel: w275 -> [w374]
      tunnel: [w375] -> w274
      tunnel: [w374] -> w273
      frame #0 {
        n126 = call "Loop Timer3"("Count(Ticks)"=w287) -> ("Tick Count(Ticks)"=w286:u32)
      }
      frame #1 {
        n127 = xnode "FPGA I/O Node"("Connector0/AO1"=w291, "Connector0/AO2"=w290) -> ()  [unwired: 2 in, 2 out]
      }
      frame #2 {
        n128 = local read "Scanning MCL"() -> (w313:bool)
        n129 = Or(x=w313, y="Start scan (MCL)") -> (x .or. y?=w308:bool)
        n130 = Not(x="Abort scan (MCL)") -> (.not. x?=w306:bool)
        n131 = And(x=w306, y=w308) -> (x .and. y?=w305:bool)
        n132 = case "Raster scan" shown="False" w305 {
          tunnel: [w314 w357] -> w310
          tunnel: "Start scan (MCL)" -> [_ w342]
          tunnel: [w314 w318] -> w294
          frame False {
            w314 = i16 0
            n133 = local write "Scanning MCL"(FALSE ("scanning")) -> ()
          }
          frame True {
            w328 = i16 0
            w327 = u64 0
            # "scan incr."
            # "freq. incr. mult."
            # "count steps"
            # "count number of cycles"
            n134 = feedback #13(w327) -> (w354:u64)
            n135 = Select(t=w327, s=w342, f=w354) -> (s? t:f=w356:u64)
            n136 = Increment(x=w356) -> (x+1=w353:u64)
            n137 = Greater?(x="Cycles per step (MCL)", y=w353) -> (0:w337:bool)
            n138 = Select(t=w353, s=w337, f=w327) -> (s? t:f=w352:u64)
            n139 = feedback-in #13(w352) -> ()
            n140 = feedback #14(w327) -> (w351:u64)
            n141 = Select(t=w327, s=w342, f=w351) -> (s? t:f=w346:u64)
            n142 = Increment(x=w346) -> (x+1=w350:u64)
            n143 = Add(x="Scan steps (MCL)", y="Scan steps (MCL)") -> (x+y=w349:u64)
            n144 = Select(t=w346, s=w337, f=w350) -> (s? t:f=w332:u64)
            n145 = Greater?(x=w349, y=w332) -> (0:w331:bool)
            n146 = Select(t=w332, s=w331, f=w327) -> (s? t:f=w347:u64)
            n147 = feedback-in #14(w347) -> ()
            n148 = Equal?(x="Scan steps (MCL)", y=w332) -> (x = y?=w336:bool)
            n149 = Greater?(x="Scan steps (MCL)", y=w346) -> (0:w345:bool)
            n150 = feedback #15(w328) -> (w348:i16)
            n151 = Select(t=w328, s=w342, f=w348) -> (s? t:f=w334:i16)
            n152 = Increment(x=w334) -> (x+1=w344:i16)
            n153 = Decrement(x=w334) -> (x-1=w343:i16)
            n154 = Select(t=w344, s=w345, f=w343) -> (s? t:f=w335:i16)
            n155 = Select(t=w334, s=w336, f=w335) -> (s? t:f=w333:i16)
            n156 = Select(t=w334, s=w337, f=w333) -> (s? t:f=w329:i16)
            n157 = Select(t=w329, s=w331, f=w328) -> (s? t:f=w330:i16)
            n158 = feedback-in #15(w330) -> ()
            n159 = feedback #16(w327) -> (w341:u64)
            n160 = Select(t=w327, s=w342, f=w341) -> (s? t:f=w316:u64)
            n161 = Increment(x=w316) -> (x+1=w338:u64)
            n162 = Select(t=w316, s=w331, f=w338) -> (s? t:f=w317:u64)
            n163 = Greater?(x="Number of scans (MCL)", y=w317) -> (0:w324:bool)
            n164 = Multiply(x="Scan freq.  increment (MCL)", y=w334) -> (x*y=w357:i16)
            n165 = Select(t=TRUE, s="Cont. Scan (MCL)", f=w324) -> (s? t:f=w323:bool)
            "Scanning MCL" <- w323
            n166 = Select(t=w317, s=w323, f=w327) -> (s? t:f=w339:u64)
            n167 = feedback-in #16(w339) -> ()
            n168 = Increment(x=w317) -> (x+1=→"Scan I (MCL)":u64)
            n169 = To Word Integer(number=w316) -> (16bit integer=w319:i16)
            n170 = Multiply(x=w319, y="Scan freq.  increment (MCL)") -> (x*y=w318:i16)
          }
        }
        n171 = Select(t=w294, s="1D or 2D Scan?", f=i16 0) -> (s? t:f=w295:i16)
        n172 = Select(t=w310, s="MCL Scan Axis", f=w295) -> (s? t:f=w311:i16)
        n173 = Select(t=w295, s="MCL Scan Axis", f=w310) -> (s? t:f=w309:i16)
        n174 = Add(x="AO2 (X)", y=w309) -> (x+y=w298:i16)
        n175 = Add(x="AO1 (Y)", y=w311) -> (x+y=w299:i16)
      }
      frame #3 {
        n176 = feedback-in #17(w380) -> ()
        n177 = feedback #17(w380) -> (w379:u32)
        n178 = Boolean To (0,1)(Boolean="+ phase (MCL)") -> (0, 1=w371:i16)
        n179 = Subtract(x=w380, y=w379) -> (x-y=w378:u32)
        n180 = Multiply(x=w371, y="Phase count adjustment (MCL)") -> (x*y=w367:i16)
        n181 = Subtract(x=w378, y=w377) -> (x-y=w359:u32)
        n182 = Subtract(x="MCL count", y=w359) -> (x-y=w369:u32)
        n183 = feedback #18(i16 0) -> (w368:i16)
        n184 = Subtract(x=w368, y=w367) -> (x-y=w366:i16)
        "MCL Relative Phase" <- w366
        n185 = feedback-in #18(w366) -> ()
        n186 = Number To Boolean Array(number=w359) -> (Boolean array=w360:bool[])
        n187 = Or Array Elements(Boolean array=w360) -> (logical OR=w358:bool)
        n188 = Boolean To (0,1)(Boolean=w358) -> (0, 1=w365:i16)
        n189 = Add(x=w369, y=w367) -> (x+y=w373:u32)
        n190 = To Unsigned Byte Integer(number=w365) -> (unsigned 8bit integer=w362:u8)
        n191 = feedback #19(u8 0) -> (w363:u8)
        n192 = Add(x=w362, y=w363) -> (x+y=w361:u8)
        "MCL Late Counter" <- w361
        n193 = feedback-in #19(w361) -> ()
      }
    }
  }
  n194 = timed-loop "APD 2 Counter" {
    tunnel: w6 -> [_]
    timing: w2 -> [_]
    timing-out: [_] -> w1
    shift-right: [w383] -> _
    shift-left: _ -> [w382]
    stop <- FALSE stop-if-true
    n195 = xnode "FPGA I/O Node"() -> ("Connector0/DIO0"=w383:bool)  [unwired: 1 in, 1 out]
    n196 = local read "APD2 int gate"() -> (w384:bool)
    n197 = Not(x=w382) -> (.not. x?=w385:bool)
    n198 = Compound Arithmetic op=OR(w383, w385, w384) -> (w386:bool)
    n199 = case shown="True" w386 {
      frame False {
      }
      frame True {
        n200 = call "Tick Count2"() -> ("Tick Count(Ticks)"=w389:u32)
        n201 = xnode ("FIFO Write")("Element"=w389, "Timeout"=0) -> ()  [unwired: 1 in, 2 out]
      }
    }
  }
  n202 = while "Green fluorescent laser interlacing (Current to IA 532 nm AOM ME amp)." {
    shift-right: [w397] -> _
    shift-left: w6 -> [w400]
    shift-right: [w394] -> _
    shift-left: i16 0 -> [w392]
    stop <- FALSE stop-if-true
    n203 = flat-sequence {
      tunnel: w400 -> [w403]
      tunnel: [w404] -> w399
      tunnel: [w403] -> w398
      tunnel: [w402] -> w393
      tunnel: w392 -> [w402]
      tunnel: [w407] -> w396
      tunnel: w399 -> [w407]
      tunnel: [w406] -> w395
      tunnel: w398 -> [w406]
      tunnel: w393 -> [w405]
      tunnel: [w420] -> w397
      tunnel: [w436] -> w394
      tunnel: w396 -> [w449]
      tunnel: w395 -> [w446]
      frame #0 {
        n204 = call "Loop Timer10"("Count(Ticks)"=w403) -> ("Tick Count(Ticks)"=w404:u32)
      }
      frame #1 {
        n205 = xnode "FPGA I/O Node"("Chassis2/Mod1/AO0"=w405) -> ()  [unwired: 1 in, 1 out]
      }
      frame #2 {
        n206 = local read "RF synth bd controls green"() -> (w411:bool)
        n207 = Subtract(x="Green interlace OFF count 2", y="Green int current ON count adj") -> (x-y=w429:u32)
        n208 = feedback-in #20(w449) -> ()
        n209 = feedback #20(w449) -> (w448:u32)
        n210 = Add(x="Green int current ON count adj", y="Green interlace ON count 2") -> (x+y=w430:u32)
        n211 = Subtract(x=w449, y=w448) -> (x-y=w447:u32)
        n212 = Subtract(x=w447, y=w446) -> (x-y=w413:u32)
        n213 = Not(x=w411) -> (.not. x?=w409:bool)
        n214 = Number To Boolean Array(number=w413) -> (Boolean array=w414:bool[])
        n215 = Boolean To (0,1)(Boolean="+ phase (GI) 2") -> (0, 1=w426:i16)
        n216 = Or Array Elements(Boolean array=w414) -> (logical OR=w412:bool)
        "GI Late?" <- w412
        n217 = Boolean To (0,1)(Boolean=w412) -> (0, 1=w419:i16)
        n218 = Multiply(x=w426, y="Phase count adjustment (GI) 2") -> (x*y=w422:i16)
        n219 = To Unsigned Word Integer(number=w419) -> (unsigned 16bit integer=w415:u16)
        n220 = feedback #21(u16 0) -> (w417:u16)
        n221 = Add(x=w415, y=w417) -> (x+y=w416:u16)
        "GI Late Counter 2" <- w416
        n222 = feedback-in #21(w416) -> ()
        n223 = feedback #22(i16 0) -> (w423:i16)
        n224 = Subtract(x=w423, y=w422) -> (x-y=w421:i16)
        "GI Relative phase 2" <- w421
        n225 = feedback-in #22(w421) -> ()
        n226 = feedback #23(TRUE) -> (w441:bool)
        n227 = case shown="2" "Operating Mode 2" {
          tunnel: [TRUE FALSE w466] -> w431
          tunnel: w441 -> [_ _ w463]
          frame 0, Default {
          }
          frame 1 {
          }
          frame 2 {
            n228 = Not(x=w463) -> (.not. x?=w465:bool)
            n229 = Select(t=w465, s="Invert GI 2", f=w463) -> (s? t:f=w466:bool)
          }
        }
        n230 = And(x=w431, y="Green FB On/Off") -> (x .and. y?=w410:bool)
        "green FB running" <- w410
        n231 = And(x=w410, y=w409) -> (x .and. y?=w408:bool)
        n232 = case shown="True" w408 {
          tunnel: "Current Out" -> [w450 _]
          tunnel: [w450 w455] -> w435
          frame False {
          }
          frame True {
            n233 = local read "Green FB Sum"() -> (w451:i16)
            n234 = call "Slower PID.vi"("process variable"=w451, "reset?"="Green FB Reset", "setpoint"="Green FB Setpoint", "PID gains (x 2^8)"="Green FB Gains", "output range"=cluster{"output high":i16, "output low":i16} {"output high"=32767, "output low"=-32768} ("Green FB output range")) -> ("output"=w459:i16)  [unwired: 10 out]
            n235 = To Long Integer(number=w459) -> (32bit integer=w452:i32)
            n236 = Add(x=w452, y=32768) -> (x+y=w454:i32)
            n237 = To Unsigned Word Integer(number=w454) -> (unsigned 16bit integer=w455:u16)
          }
        }
        n238 = Not(x=w441) -> (.not. x?=w438:bool)
        n239 = Select(t=w430, s=w438, f=w429) -> (s? t:f=w443:u32)
        n240 = Subtract(x=w443, y=w413) -> (x-y=w424:u32)
        n241 = Add(x=w424, y=w422) -> (x+y=w420:u32)
        n242 = feedback-in #23(w438) -> ()
        n243 = Boolean To (0,1)(Boolean=w431) -> (0, 1=w437:i16)
        n244 = To Unsigned Word Integer(number=w437) -> (unsigned 16bit integer=w434:u16)
        n245 = Multiply(x=w434, y=w435) -> (x*y=w436:u16)
      }
    }
  }
  n246 = timed-loop "APD 1 Counter" {
    tunnel: w6 -> [_]
    shift-right: [w469] -> _
    shift-left: _ -> [w471]
    timing: w4 -> [_]
    timing-out: [_] -> w3
    stop <- FALSE stop-if-true
    n247 = xnode "FPGA I/O Node"() -> ("Connector0/DIO0"=w469:bool)  [unwired: 1 in, 1 out]
    n248 = local read "APD1 int gate"() -> (w470:bool)
    n249 = Not(x=w471) -> (.not. x?=w468:bool)
    n250 = Compound Arithmetic op=OR(w469, w468, w470) -> (w467:bool)
    n251 = case shown="True" w467 {
      frame False {
      }
      frame True {
        n252 = call "Tick Count"() -> ("Tick Count(Ticks)"=w474:u32)
        n253 = xnode ("FIFO Write")("Element"=w474, "Timeout"=0) -> ()  [unwired: 1 in, 2 out]
      }
    }
  }
  n254 = while "RF synth board interlacing timing loop" {
    tunnel: w6 -> [_]
    stop <- FALSE stop-if-true
    # "This loop is stalled until the RF FIFO get a value. With this method we gain additional delay time (because  we allow the rest of the main RF loop to procede while this loop waits to send the switch signals - a form of parallelism). This helps to simplify the main RF code. \n\nThe code also allow optimal interlacing while also controlling trap RF phase. \n\nNote: a lot of work has gone into optimizing these methods and it is unclear how they can be made any faster or better than this (many failed tries). Right now there is essentially ~4 ticks (~90 ns ns) of imperfection in the switching from trap 1 to trap 2. ~2 ticks of no RF (phase reset) then ~2 ticks of trap 2 with the wrong amplitude (T1 amplitude). The total ticks is 200, so not a big error.\n\nPhase can be precisely set for each trap. Phase reset and switching, has similar delays as fsk frequency switching. And phase reset and phase offset changes are also not simultaneous. So we can't perfectly line everything up.\n\nIf you start from amp zero though (as for trap 1), the on switch is perfect. Likewise the off is perfect for trap 2. \n\nThe green laser switching is also perfect because of its reduced duty cycle and delays in fsk switching between 80 and 0 MHz."
    n255 = xnode ("FIFO Read")("Timeout"=-1) -> ("Element"=w523:u16, "FIFO Out"=w519:refnum<k21>)  [unwired: 1 in, 1 out]
    n256 = Equal To 0?(x=w523) -> (x = 0?=w520:bool)
    n257 = Not(x=w520) -> (.not. x?=w477:bool)
    n258 = flat-sequence "BD 1 and 2 RF phase and amplitude switching" {
      tunnel: w477 -> [_]
      tunnel: w512 -> [w627]
      tunnel: w511 -> [w626]
      tunnel: w510 -> [w625]
      tunnel: w509 -> [w624]
      tunnel: w508 -> [w623]
      tunnel: w507 -> [w622]
      tunnel: w506 -> [w621]
      tunnel: w505 -> [w620]
      tunnel: w503 -> [w619]
      tunnel: w502 -> [w618]
      tunnel: w501 -> [w617]
      tunnel: w499 -> [w615]
      tunnel: w498 -> [w614]
      tunnel: w497 -> [w613]
      tunnel: w500 -> [w616]
      tunnel: w504 -> [w612]
      tunnel: w496 -> [w651]
      tunnel: w495 -> [w650]
      tunnel: w494 -> [w649]
      tunnel: w493 -> [w648]
      tunnel: w492 -> [w647]
      tunnel: w491 -> [w646]
      tunnel: w490 -> [w645]
      tunnel: w489 -> [w644]
      tunnel: w488 -> [w643]
      tunnel: w486 -> [w642]
      tunnel: w485 -> [w641]
      tunnel: w484 -> [w640]
      tunnel: w483 -> [w639]
      tunnel: w482 -> [w638]
      tunnel: w481 -> [w637]
      tunnel: w487 -> [w636]
      frame #0 {
        # "Delay to align amp/frequency switching depending on the method used.\n\nCan also give enough time to do the parallel amplitude calculations"
        n259 = call "Wait2"("Count(Ticks)"="Amp switch delay") -> ()  [unwired: 1 out]
      }
      frame #1 {
        w607 = TRUE ("Connector1/DIO30")
        # "make phase offset and phase reset active with buffer transfer"
        n260 = xnode "FPGA I/O Node"("Connector1/DIO29"=w607, "Connector1/DIO30"=w607) -> ()  [unwired: 2 in, 2 out]
      }
      frame #2 {
        w608 = FALSE ("Connector1/DIO15")
        # "write phase restart to buffer and reset udclk"
        n261 = xnode "FPGA I/O Node"("Connector1/DIO29"=w608, "Connector1/DIO30"=w608, "Connector1/DIO15"=FALSE ("Connector1/DIO14")) -> ()  [unwired: 3 in, 3 out]
      }
      frame #3 {
        w610 = TRUE ("Connector1/DIO15")
        # "make phase restart active"
        # "reset WR"
        n262 = xnode "FPGA I/O Node"("Connector1/DIO15"=w610, "Connector1/DIO29"=w610, "Connector1/DIO30"=w610) -> ()  [unwired: 3 in, 3 out]
      }
      frame #4 {
        w611 = FALSE ("Connector1/DIO30")
        # "Address"
        # "set amp byte 1, and reset udclk"
        n263 = xnode "FPGA I/O Node"("Connector1/DIO0"=w627, "Connector1/DIO1"=w626, "Connector1/DIO2"=w625, "Connector1/DIO3"=w624, "Connector1/DIO4"=w623, "Connector1/DIO5"=w622, "Connector1/DIO6"=w621, "Connector1/DIO7"=w620, "Connector1/DIO8"=TRUE, "Connector1/DIO9"=FALSE, "Connector1/DIO10"=FALSE, "Connector1/DIO11"=FALSE, "Connector1/DIO12"=FALSE, "Connector1/DIO13"=TRUE, "Connector1/DIO20"=w612, "Connector1/DIO21"=w619, "Connector1/DIO22"=w618, "Connector1/DIO23"=w617, "Connector1/DIO24"=w616, "Connector1/DIO25"=w615, "Connector1/DIO26"=w614, "Connector1/DIO27"=w613, "Connector1/DIO30"=w611, "Connector1/DIO29"=w611) -> ()  [unwired: 24 in, 24 out]
      }
      frame #5 {
        # "write amp byte 1 to buffer"
        n264 = xnode "FPGA I/O Node"("Connector1/DIO15"=FALSE ("Connector1/DIO14")) -> ()  [unwired: 1 in, 1 out]
      }
      frame #6 {
        # "reset WR"
        n265 = xnode "FPGA I/O Node"("Connector1/DIO15"=TRUE) -> ()  [unwired: 1 in, 1 out]
      }
      frame #7 {
        # "Address"
        # "set amp byte 2"
        n266 = xnode "FPGA I/O Node"("Connector1/DIO0"=w651, "Connector1/DIO1"=w650, "Connector1/DIO2"=w649, "Connector1/DIO3"=w648, "Connector1/DIO4"=w647, "Connector1/DIO5"=w646, "Connector1/DIO6"=w645, "Connector1/DIO7"=w644, "Connector1/DIO8"=TRUE, "Connector1/DIO9"=FALSE, "Connector1/DIO10"=FALSE, "Connector1/DIO11"=FALSE, "Connector1/DIO12"=TRUE, "Connector1/DIO13"=FALSE, "Connector1/DIO20"=w643, "Connector1/DIO21"=w636, "Connector1/DIO22"=w642, "Connector1/DIO23"=w641, "Connector1/DIO24"=w640, "Connector1/DIO25"=w639, "Connector1/DIO26"=w638, "Connector1/DIO27"=w637) -> ()  [unwired: 22 in, 22 out]
      }
      frame #8 {
        # "write amp byte 2"
        n267 = xnode "FPGA I/O Node"("Connector1/DIO15"=FALSE ("Connector1/DIO14")) -> ()  [unwired: 1 in, 1 out]
      }
      frame #9 {
        w659 = TRUE ("Connector1/DIO15")
        # "transfer amp bytes 1 and 2 and reset WR"
        n268 = xnode "FPGA I/O Node"("Connector1/DIO29"=w659, "Connector1/DIO30"=w659, "Connector1/DIO15"=TRUE ("Connector1/DIO14")) -> ()  [unwired: 3 in, 3 out]
      }
      frame #10 {
        w661 = FALSE ("Connector1/DIO14")
        # "reset udclk"
        n269 = xnode "FPGA I/O Node"("Connector1/DIO29"=w661, "Connector1/DIO30"=w661) -> ()  [unwired: 2 in, 2 out]
      }
    }
    n270 = flat-sequence "FSK BD 1 (trap X)" {
      tunnel: w477 -> [w525]
      tunnel: [w525] -> w480
      tunnel: w480 -> [w526]
      frame #0 {
        n271 = call "Wait"("Count(Ticks)"="BD 1 Delay (ticks)") -> ()  [unwired: 1 out]
      }
      frame #1 {
        # "switch frequency"
        n272 = xnode "FPGA I/O Node"("Connector1/DIO36"=w526) -> ()  [unwired: 1 in, 1 out]
      }
    }
    n273 = flat-sequence "FSK BD 2 (trap Y or green laser AOM)" {
      tunnel: w477 -> [w663]
      tunnel: [w663] -> w522
      tunnel: w522 -> [w664]
      frame #0 {
        n274 = call "Wait3"("Count(Ticks)"="BD 2 Delay (Ticks)") -> ()  [unwired: 1 out]
      }
      frame #1 {
        # "switch frequency"
        n275 = xnode "FPGA I/O Node"("Connector1/DIO37"=w664) -> ()  [unwired: 1 in, 1 out]
      }
    }
    n276 = xnode ("FIFO Read")("Timeout"=-1, "FIFO In"=w519) -> ("Element"=w514:u16, "FIFO Out"=w518:refnum<k21>)  [unwired: 1 out]
    n277 = xnode ("FIFO Read")("Timeout"=-1, "FIFO In"=w518) -> ("Element"=w513:u16)  [unwired: 2 out]
    n278 = node-c288() -> (w516:T7)  [unwired: 1 in]
    n279 = timed-loop "Convert amplitude words to bits" {
      timing: w516 -> [_]
      timing-out: [_] -> w515
      tunnel: w514 -> [w583]
      tunnel: w513 -> [w582]
      tunnel: [w559] -> w512
      tunnel: [w558] -> w511
      tunnel: [w557] -> w510
      tunnel: [w556] -> w509
      tunnel: [w555] -> w508
      tunnel: [w554] -> w507
      tunnel: [w553] -> w506
      tunnel: [w552] -> w505
      tunnel: [w551] -> w504
      tunnel: [w550] -> w503
      tunnel: [w549] -> w502
      tunnel: [w548] -> w501
      tunnel: [w547] -> w500
      tunnel: [w546] -> w499
      tunnel: [w545] -> w498
      tunnel: [w544] -> w497
      tunnel: [w543] -> w496
      tunnel: [w542] -> w495
      tunnel: [w541] -> w494
      tunnel: [w540] -> w493
      tunnel: [w539] -> w492
      tunnel: [w538] -> w491
      tunnel: [w537] -> w490
      tunnel: [w536] -> w489
      tunnel: [w535] -> w488
      tunnel: [w534] -> w487
      tunnel: [w533] -> w486
      tunnel: [w532] -> w485
      tunnel: [w531] -> w484
      tunnel: [w530] -> w483
      tunnel: [w529] -> w482
      tunnel: [w528] -> w481
      stop <- TRUE stop-if-true
      # "Board 1 Data"
      # "Board 2 Data"
      # "Board 1 Data"
      # "Board 2 Data"
      n280 = Split Number(x=w583) -> (hi(x)=w581:u8, lo(x)=w561:u8)
      n281 = Split Number(x=w582) -> (hi(x)=w580:u8, lo(x)=w560:u8)
      n282 = Number To Boolean Array(number=w581) -> (Boolean array=w601:bool[])
      n283 = Number To Boolean Array(number=w580) -> (Boolean array=w592:bool[])
      n284 = Index Array(array=w601, index=7) -> (element=w559:bool)
      n285 = Index Array(array=w601, index=6) -> (element=w558:bool)
      n286 = Index Array(array=w601, index=5) -> (element=w557:bool)
      n287 = Index Array(array=w601, index=4) -> (element=w556:bool)
      n288 = Index Array(array=w601, index=3) -> (element=w555:bool)
      n289 = Index Array(array=w601, index=2) -> (element=w554:bool)
      n290 = Index Array(array=w601, index=1) -> (element=w553:bool)
      n291 = Index Array(array=w601, index=0) -> (element=w552:bool)
      n292 = Index Array(array=w592, index=7) -> (element=w551:bool)
      n293 = Index Array(array=w592, index=6) -> (element=w550:bool)
      n294 = Index Array(array=w592, index=5) -> (element=w549:bool)
      n295 = Index Array(array=w592, index=4) -> (element=w548:bool)
      n296 = Index Array(array=w592, index=3) -> (element=w547:bool)
      n297 = Index Array(array=w592, index=2) -> (element=w546:bool)
      n298 = Index Array(array=w592, index=1) -> (element=w545:bool)
      n299 = Index Array(array=w592, index=0) -> (element=w544:bool)
      n300 = Number To Boolean Array(number=w561) -> (Boolean array=w579:bool[])
      n301 = Number To Boolean Array(number=w560) -> (Boolean array=w570:bool[])
      n302 = Index Array(array=w579, index=7) -> (element=w543:bool)
      n303 = Index Array(array=w579, index=6) -> (element=w542:bool)
      n304 = Index Array(array=w579, index=5) -> (element=w541:bool)
      n305 = Index Array(array=w579, index=4) -> (element=w540:bool)
      n306 = Index Array(array=w579, index=3) -> (element=w539:bool)
      n307 = Index Array(array=w579, index=2) -> (element=w538:bool)
      n308 = Index Array(array=w579, index=1) -> (element=w537:bool)
      n309 = Index Array(array=w579, index=0) -> (element=w536:bool)
      n310 = Index Array(array=w570, index=7) -> (element=w535:bool)
      n311 = Index Array(array=w570, index=6) -> (element=w534:bool)
      n312 = Index Array(array=w570, index=5) -> (element=w533:bool)
      n313 = Index Array(array=w570, index=4) -> (element=w532:bool)
      n314 = Index Array(array=w570, index=3) -> (element=w531:bool)
      n315 = Index Array(array=w570, index=2) -> (element=w530:bool)
      n316 = Index Array(array=w570, index=1) -> (element=w529:bool)
      n317 = Index Array(array=w570, index=0) -> (element=w528:bool)
    }
    n318 = node-c288(w515) -> ()
  }
  n319 = while "APD 1 Gating" {
    shift-right: [w668] -> _
    shift-left: w6 -> [w673]
    shift-right: [w667] -> _
    shift-left: w8 -> [w665]
    stop <- FALSE stop-if-true
    n320 = flat-sequence {
      tunnel: w673 -> [w676]
      tunnel: [w677] -> w671
      tunnel: [w676] -> w669
      tunnel: [w675] -> w666
      tunnel: w665 -> [w675]
      tunnel: [w680] -> w672
      tunnel: w671 -> [w680]
      tunnel: [w679] -> w670
      tunnel: w669 -> [w679]
      tunnel: w666 -> [w678]
      tunnel: [w700] -> w668
      tunnel: w672 -> [w714]
      tunnel: w670 -> [w711]
      tunnel: [w682] -> w667
      frame #0 {
        n321 = call "Loop Timer4"("Count(Ticks)"=w676) -> ("Tick Count(Ticks)"=w677:u32)
      }
      frame #1 {
        # "Signal maybe then sent through \na transistor before APD"
        n322 = xnode "FPGA I/O Node"("Connector1/DIO33"=w678) -> ()  [unwired: 1 in, 1 out]
        "APD1 int gate" <- w678
      }
      frame #2 {
        n323 = feedback #24(TRUE) -> (w706:bool)
        n324 = feedback-in #25(w714) -> ()
        n325 = feedback #25(w714) -> (w713:u32)
        n326 = Not(x=w706) -> (.not. x?=w703:bool)
        n327 = feedback-in #24(w703) -> ()
        n328 = Subtract(x=w714, y=w713) -> (x-y=w712:u32)
        n329 = Select(t="APD Gate ON Count", s=w703, f="APD Gate OFF Count") -> (s? t:f=w708:u16)
        n330 = Subtract(x=w712, y=w711) -> (x-y=w688:u32)
        n331 = Subtract(x=w708, y=w688) -> (x-y=w699:u32)
        n332 = Number To Boolean Array(number=w688) -> (Boolean array=w689:bool[])
        n333 = Or Array Elements(Boolean array=w689) -> (logical OR=w687:bool)
        n334 = Boolean To (0,1)(Boolean="+ phase (APD 1 Gate)") -> (0, 1=w697:i16)
        n335 = Boolean To (0,1)(Boolean=w687) -> (0, 1=w694:i16)
        n336 = Multiply(x=w697, y="Phase count adjustment (APD 1 Gate)") -> (x*y=w695:i16)
        n337 = To Unsigned Byte Integer(number=w694) -> (unsigned 8bit integer=w691:u8)
        n338 = Add(x=w699, y=w695) -> (x+y=w700:u32)
        n339 = feedback #26(i16 0) -> (w702:i16)
        n340 = Subtract(x=w702, y=w695) -> (x-y=w701:i16)
        "APD 1 Gate Relative Phase" <- w701
        n341 = feedback-in #26(w701) -> ()
        n342 = feedback #27(u8 0) -> (w692:u8)
        n343 = Add(x=w691, y=w692) -> (x+y=w690:u8)
        "APD 1 Gate Late Counter" <- w690
        n344 = feedback-in #27(w690) -> ()
        n345 = local read "Green long-scale interlacing"() -> (w681:bool)
        n346 = case shown="2" "APD Gate Operating Mode" {
          tunnel: [TRUE FALSE w736] -> w684
          tunnel: w706 -> [_ _ w736]
          frame 0, Default {
          }
          frame 1 {
          }
          frame 2 {
          }
        }
        n347 = Not(x=w684) -> (.not. x?=w685:bool)
        n348 = Select(t=w685, s="Invert APD Gate", f=w684) -> (s? t:f=w683:bool)
        n349 = case shown="True" w681 {
          tunnel: w683 -> [w715 w723]
          tunnel: [w715 w724] -> w682
          frame False {
          }
          frame True {
            n350 = local read "Number of ON cycles"() -> (w717:i16)
            n351 = local read "Number of OFF cycles"() -> (w719:i16)
            n352 = feedback #28(i16 1) -> (w730:i16)
            n353 = Increment(x=w730) -> (x+1=w729:i16)
            n354 = feedback #29(w717) -> (w716:i16)
            n355 = Greater?(x=w716, y=w730) -> (0:w725:bool)
            n356 = Select(t=w729, s=w725, f=i16 1) -> (s? t:f=w727:i16)
            n357 = feedback-in #28(w727) -> ()
            n358 = feedback #30(TRUE) -> (w722:bool)
            n359 = Not(x=w722) -> (.not. x?=w721:bool)
            n360 = Select(t=w722, s=w725, f=w721) -> (s? t:f=w720:bool)
            n361 = feedback-in #30(w720) -> ()
            n362 = Select(t=w717, s=w720, f=w719) -> (s? t:f=w718:i16)
            n363 = feedback-in #29(w718) -> ()
            n364 = case shown="True" w720 {
              tunnel: [FALSE w733] -> w724
              tunnel: w723 -> [_ w733]
              frame False {
              }
              frame True {
              }
            }
          }
        }
      }
    }
  }
  n365 = while "Trap RF control, main calculations (raster scanning, intensity and position feedback, phase control etc) with primary timing trigger" {
    shift-right: [w751] -> _
    shift-left: w6 -> [w750]
    shift-right: [w749] -> _
    shift-left: FALSE ("Swap F1 and F2") -> [w748]
    shift-right: [w744] -> _
    shift-left: u16 0 ("BD 1 Amplitude 3") -> [w741]
    shift-right: [w743] -> _
    shift-left: u16 0 ("BD 2 Amplitude 3") -> [w739]
    shift-right: [w738] -> _
    shift-left: u64 0 -> [w737]
    stop <- FALSE stop-if-true
    n366 = flat-sequence {
      tunnel: w748 -> [w757]
      tunnel: w750 -> [w754]
      tunnel: [w757] -> w747
      tunnel: [w753] -> w746
      tunnel: [w754] -> w745
      tunnel: [w756] -> w742
      tunnel: w741 -> [w756]
      tunnel: [w755] -> w740
      tunnel: w739 -> [w755]
      tunnel: [w768] -> w751
      tunnel: [w767] -> w749
      tunnel: w747 -> [w766]
      tunnel: w746 -> [w765]
      tunnel: w745 -> [w764]
      tunnel: [w763] -> w744
      tunnel: [w762] -> w743
      tunnel: w742 -> [w761]
      tunnel: w740 -> [w760]
      tunnel: [w759] -> w738
      tunnel: w737 -> [w758]
      frame #0 {
        n367 = call "Loop Timer2"("Count(Ticks)"=w754) -> ("Tick Count(Ticks)"=w753:u32)
      }
      frame #1 {
        n368 = flat-sequence {
          tunnel: w766 -> [w776]
          tunnel: w761 -> [w770]
          tunnel: w760 -> [w769]
          tunnel: [w836] -> w768
          tunnel: [w848] -> w767
          tunnel: w765 -> [w842]
          tunnel: w764 -> [w839]
          tunnel: [w787] -> w763
          tunnel: [w786] -> w762
          tunnel: [w778] -> w759
          tunnel: w758 -> [w777]
          frame #0 {
            w771 = -1 ("Timeout")
            # "Operation when you need a long delay for either X or Y to synchonize AOD light out phase (> ~100 ticks)\nor want shorter trap ON timing. Puts some of the delay timing in parallel with the later computations."
            # "Trigger the external loop by sending the boolean FSK value through a FIFO.\nTiming is precise."
            n369 = Boolean To (0,1)(Boolean=w776) -> (0, 1=w775:i16)
            n370 = To Unsigned Word Integer(number=w775) -> (unsigned 16bit integer=w774:u16)
            n371 = xnode ("FIFO Method Node")("Element"=w774, "Timeout"=w771) -> ("FIFO Out"=w773:refnum<k21>)  [unwired: 1 in, 1 out]
            n372 = xnode ("FIFO Method Node")("Element"=w770, "Timeout"=w771, "FIFO In"=w773) -> ("FIFO Out"=w772:refnum<k21>)  [unwired: 1 out]
            n373 = xnode ("FIFO Method Node")("Element"=w769, "Timeout"=w771, "FIFO In"=w772) -> ()  [unwired: 2 out]
          }
          frame #1 {
            # "Just counts, wraps around, 8 bit"
            # "Which trap cycle"
            # "Only save the 3rd set's amp in the loop"
            # "If this is NOT set 3 AND NOT (RF synth controls green AND green FB running)\nthen use this sets amp value (otherwise keep the green feedback value)"
            # "Just flips back and forth."
            # "If interlacing is off, this is which cycle to use."
            # "Keep track of trap cycles (trap 1, 2, 3...)"
            # "This is the prior cycle's on time"
            # "increment timing\nindex, reset to 0 if \nend of matrix"
            # "Reset to begginning (1) when number of cycles reached."
            # "timing index"
            # "build byte stacks for writing data\n(must correspond to addresses array constant)"
            # "Timing housekeeping"
            # "Adjust phase if late\n(maintains constant phase relationship between cycles)"
            n374 = feedback #31(u8 0 ("t")) -> (w845:u8)
            n375 = Increment(x=w845) -> (x+1=w884:u8)
            n376 = Increment(x="Number Interlace Cycles") -> (x+1=w879:u8)
            n377 = Equal?(x=w884, y=w879) -> (x = y?=w886:bool)
            n378 = Select(t=u8 1, s=w886, f=w884) -> (s? t:f=w844:u8)
            n379 = feedback-in #31(w844) -> ()
            n380 = Increment(x=w844) -> (x+1=w881:u8)
            n381 = Equal?(x=w881, y=w879) -> (x = y?=w882:bool)
            n382 = Select "This cycle"(t=u8 1, s=w882, f=w881) -> (s? t:f=w878:u8)
            n383 = Select(t=w878, s="Interlace ON/OFF", f="Interlace Off Parameters") -> (s? t:f=w797:u8)
            n384 = feedback-in #32(w842) -> ()
            n385 = feedback #32(w842) -> (w841:u32)
            n386 = Select(t=w844, s="Interlace ON/OFF", f="Interlace Off Parameters") -> (s? t:f=w877:u8)
            n387 = Subtract(x=w842, y=w841) -> (x-y=w840:u32)
            n388 = Subtract "The error"(x=w840, y=w839) -> (x-y=w823:u32)
            n389 = case shown="1, Default" w877 {
              tunnel: ["DIO count 1 (ticks)" "DIO count 2 (ticks)" "DIO count 3 (ticks)"] -> w838
              frame 1, Default {
              }
              frame 2 {
              }
              frame 3 {
              }
            }
            n390 = Number To Boolean Array(number=w823) -> (Boolean array=w824:bool[])
            n391 = Or Array Elements(Boolean array=w824) -> (logical OR=w822:bool)
            n392 = Boolean To (0,1)(Boolean=w822) -> (0, 1=w829:i16)
            n393 = To Unsigned Byte Integer(number=w829) -> (unsigned 8bit integer=w826:u8)
            n394 = feedback #33(u8 0) -> (w827:u8)
            n395 = Add(x=w826, y=w827) -> (x+y=w825:u8)
            "DIO Late Counter" <- w825
            n396 = feedback-in #33(w825) -> ()
            n397 = Subtract(x=w838, y=w823) -> (x-y=w837:u32)
            n398 = disable-structure shown="Disabled" {
              disable-tunnel: [w890 _] -> w821
              disable-tunnel: w797 -> [w887 _]
              frame Disabled {
                n399 = feedback #34(i64 0 ("y")) -> (w889:i64)
                n400 = case "Synchronize trap oscillations - always begin/end with trap 1" shown="1, Default" w887 {
                  tunnel: [w891 w892 w893] -> w890
                  tunnel: w889 -> [w891 w892 _]
                  frame 2 {
                  }
                  frame 3 {
                  }
                  frame 1, Default {
                    n401 = Or(x="Osc traps", y="Initiate trap osc") -> (x .or. y?=w895:bool)
                    n402 = case "Trap sine oscillation (or whatever pattern is stored in memory)" shown="True" w895 {
                      tunnel: [i64 0 ("y") w899] -> w893
                      tunnel: "Initiate trap osc" -> [_ w902]
                      frame False {
                      }
                      frame True {
                        w906 = u16 0
                        w904 = -1
                        n403 = local write "Initiate trap osc"(FALSE ("Initiate trap osc")) -> ()
                        n404 = feedback #35(w906) -> (w908:u16)
                        n405 = Select(t=w906, s=w902, f=w908) -> (s? t:f=w907:u16)
                        n406 = Greater Or Equal?(x=w907, y="Trap osc period (pts)") -> (x >= y?=w913:bool)
                        n407 = Or(x=w902, y=w913) -> (x .or. y?=w914:bool)
                        n408 = Select(t=u16 0, s=w914, f=w907) -> (s? t:f=w898:u16)
                        n409 = feedback #36(w904) -> (w905:i32)
                        n410 = Select(t=w904, s=w902, f=w905) -> (s? t:f=w903:i32)
                        n411 = Increment(x=w903) -> (x+1=w910:i32)
                        n412 = Equal?(x=w898, y=u16 0) -> (x = y?=w911:bool)
                        n413 = Increment(x=w898) -> (x+1=w918:u16)
                        n414 = feedback-in #35(w918) -> ()
                        n415 = Select(t=w910, s=w911, f=w903) -> (s? t:f=w909:i32)
                        n416 = feedback-in #36(w909) -> ()
                        n417 = case shown="False" "Osc trap cont." {
                          tunnel: w909 -> [w922 _]
                          frame False {
                            n418 = Greater Or Equal?(x=w922, y="N trap osc periods") -> (x >= y?=w920:bool)
                            n419 = Not(x=w920) -> (.not. x?=w919:bool)
                            n420 = local write "Osc traps"(w919) -> ()
                          }
                          frame True {
                          }
                        }
                        n421 = xnode ("Memory Read")("Address"=w898, "Memory In"=refnum<k21> "Trap osc memory") -> ("Data"=w899:i64)  [unwired: 1 out]
                      }
                    }
                  }
                }
                n422 = feedback-in #34(w890) -> ()
              }
              frame Enabled {
              }
            }
            n423 = local read "green FB running"() -> (w810:bool)
            n424 = And(x=w810, y="RF synth bd controls green") -> (x .and. y?=w809:bool)
            n425 = case shown="1, Default" w797 {
              tunnel: [w1049 w1285 "BD 1 Frequency 3"] -> w874
              tunnel: [w1090 w1284 w1306] -> w813
              tunnel: ["BD 2 Amplitude 1" "BD 2 Amplitude 2" w1305] -> w805
              tunnel: [w1046 w1281 "BD 1 Amplitude 3"] -> w787
              tunnel: "FB Gains" -> [w1067 w1291 _]
              tunnel: "FB output range" -> [w1068 w1290 _]
              tunnel: w821 -> [w1065 w1288 _]
              tunnel: "BD 2 Frequency 1" -> [w1062 _ _]
              tunnel: "BD 2 Frequency 2" -> [_ w1284 _]
              tunnel: "BD 2 Frequency 3" -> [_ _ w1306]
              tunnel: w809 -> [_ _ w1304]
              tunnel: [w1049 w1282 w1303] -> w778
              tunnel: w777 -> [w1048 w1282 w1303]
              frame 1, Default {
                w1081 = fxp<+/-,24,9> 0.0 ("AI1 X Set 2")
                w1075 = u16 0
                w1088 = u64 0 ("f")
                # "Changed by Ronen - correction \nby PID is now implemented not on \nthe Base BD1 frequency but on the last\nfrequency sent."
                # "Added by Ronen -\nUpper and Lower \nLimits for the FB \ngenerated frequency\nto avoid losing bead \nwhen tether breaks"
                # "Explanation of raster scanning:\n1. Cycles: increment counter by 1 every time interlace cycle returns to trap 1. As long as \n  Cycle per Step is larger than counter, keep incrementing counter and do not change step counter.\n  Once counter is equal to Cycles per step, zero counter and increment step counter.\n2. Steps: Increments up every time cycles counter equals cycles per step. Performs the following:\n- To determine DIRECTION of frequency change:  If ScanstepX2 is EQUAL to step counter (full for-back scan finished)\n   frequency increment is set to zero, AND step counter is set to zero. \n   Otherwise: if no change to step counter (because cycleperstep>cycle counter), then no change to frequency\n   increment. \n   If step counter has changed (cycleperstep=cycle counter), then need to figure out direction of frequency change:\n   if step counter is EQUAL to Scansteps: No change to frequency increment\n   Otherwise: If scan steps > step counter - 1 (forward scan NOT completed): increment frequency by 1\n                       If scan steps equal or smaller than step counter -1 (forward scan completed): increment frequency by -1\n\n3. Scans: Increment scan counter every time step counter equals 2Xscan steps (full for-back scan completed)\n    if number of scans > scan counter: Send TRUE to scanning, continue scan\n    if number of scans = scan counter: Send FALSE to Scanning, Scan finished.\n\n  The wire with the asterik can be used as the index for getting the mirror positions in the offset scan."
                # "This signal integration happens no matter what\nso that correct setpoints can be chosen before \nturning on the FB."
                # "Trap 1"
                n426 = local read "AI1 X Set 2"() -> (w1060:fxp<+/-,16,1>)
                n427 = local read "AI1 X Set 1"() -> (w1078:fxp<+/-,16,1>)
                n428 = local read "Scanning"() -> (w1091:bool)
                n429 = Multiply(x=w1060, y="B factor") -> (x*y=w1058:fxp<+/-,48,17>)
                n430 = Or(x=w1091, y="Start scan") -> (x .or. y?=w1043:bool)
                n431 = case shown="True" "Diff FB Measurement?" {
                  tunnel: w1058 -> [w1181 w1190]
                  tunnel: w1078 -> [w1180 w1191]
                  tunnel: [w1178 w1182] -> w1079
                  frame False {
                    n432 = Select(t=w1180, s="Trap Pos FB Monitor T1 or T2", f=w1181) -> (s? t:f=w1178:fxp<+/-,48,17>)
                  }
                  frame True {
                    n433 = Subtract(x=w1191, y=w1190) -> (x-y=w1183:fxp<+/-,48,17>)
                    n434 = Not(x="Negate Diff?") -> (.not. x?=w1189:bool)
                    n435 = Boolean To (0,1)(Boolean="Negate Diff?") -> (0, 1=w1187:i16)
                    n436 = Boolean To (0,1)(Boolean=w1189) -> (0, 1=w1188:i16)
                    n437 = Negate(x=w1187) -> (-x=w1186:i16)
                    n438 = Add(x=w1186, y=w1188) -> (x+y=w1184:i16)
                    n439 = Multiply(x=w1184, y=w1183) -> (x*y=w1182:fxp<+/-,63,32>)
                  }
                }
                n440 = feedback #37(w1075) -> (w1074:u16)
                n441 = Increment(x=w1074) -> (x+1=w1076:u16)
                n442 = Greater Or Equal?(x=w1076, y="Trap Pos FB Int Count") -> (x >= y?=w1047:bool)
                n443 = Select(t=w1075, s=w1047, f=w1076) -> (s? t:f=w1077:u16)
                n444 = feedback-in #37(w1077) -> ()
                n445 = feedback #38(w1081) -> (w1080:fxp<+/-,24,9>)
                n446 = Add(x=w1079, y=w1080) -> (x+y=w1073:fxp<+/-,24,9>)
                n447 = Select(t=w1081, s=w1047, f=w1073) -> (s? t:f=w1084:fxp<+/-,24,9>)
                n448 = feedback-in #38(w1084) -> ()
                n449 = case "Trap 1 X intensity feedback" shown="True" "FB On/Off Set 1" {
                  tunnel: "BD 1 Amplitude 1" -> [w1273 _]
                  tunnel: [w1273 w1277] -> w1046
                  tunnel: w1068 -> [_ w1274]
                  tunnel: w1067 -> [_ w1275]
                  frame False {
                  }
                  frame True {
                    n450 = local read "AI2 Y Sum Set 1"() -> (w1278:i16)
                    n451 = call "Slower PID.vi"("process variable"=w1278, "reset?"="FB Reset Set 1", "setpoint"="FB Setpoint Set 1", "PID gains (x 2^8)"=w1275, "output range"=w1274) -> ("output"=w1279:i16)  [unwired: 10 out]
                    n452 = To Unsigned Word Integer(number=w1279) -> (unsigned 16bit integer=w1277:u16)
                  }
                }
                "BD1 amplitude 1 out" <- w1046
                n453 = Divide(x=w1073, y="Trap Pos FB Int Count") -> (x/y=w1044:fxp<+/-,16,1>)
                n454 = case "For raster scanning" shown="True" w1043 {
                  tunnel: [u64 0 w1121] -> w1045
                  tunnel: [FALSE w1109] -> w1038
                  tunnel: [i16 0 w1108] -> w1039
                  tunnel: w1044 -> [_ w1107]
                  tunnel: "Start scan" -> [_ w1101]
                  frame False {
                    n455 = local write "Scanning"(FALSE ("scanning")) -> ()
                  }
                  frame True {
                    w1115 = u64 0
                    # "Changed by RG, to introduce force\ndependent stopping of the raster scan \nand manual stopping"
                    # "count number of cycles"
                    n456 = feedback #39(w1115) -> (w1118:u64)
                    n457 = Select(t=w1115, s=w1101, f=w1118) -> (s? t:f=w1120:u64)
                    n458 = Increment(x=w1120) -> (x+1=w1113:u64)
                    n459 = Equal?(x=i16 1, y=w1113) -> (x = y?=w1111:bool)
                    n460 = And(x="Abort scan", y=w1111) -> (x .and. y?=w1109:bool)
                    n461 = Greater?(x="Cycles per step", y=w1113) -> (0:w1116:bool)
                    n462 = Select(t=w1113, s=w1116, f=w1115) -> (s? t:f=w1117:u64)
                    n463 = feedback-in #39(w1117) -> ()
                    n464 = Greater?(x=w1107, y="Raster setpoint") -> (0:w1104:bool)
                    n465 = And(x=w1104, y="Raster to target force") -> (x .and. y?=w1102:bool)
                    n466 = case shown="False" w1109 {
                      tunnel: [w1128 i16 0] -> w1121
                      tunnel: w1101 -> [w1153 _]
                      tunnel: w1116 -> [w1146 _]
                      tunnel: w1115 -> [w1136 _]
                      tunnel: [w1130 FALSE] -> w1110
                      tunnel: [w1126 w1164] -> w1108
                      tunnel: [w1129 w1165] -> w1105
                      frame False {
                        w1137 = i64 0
                        # "scan incr."
                        # "freq. incr. mult."
                        # "count steps"
                        n467 = feedback #40(w1136) -> (w1161:u64)
                        n468 = Select(t=w1136, s=w1153, f=w1161) -> (s? t:f=w1129:u64)
                        n469 = Increment(x=w1129) -> (x+1=w1160:u64)
                        n470 = Add(x="Scan steps", y="Scan steps") -> (x+y=w1159:u64)
                        n471 = Select(t=w1129, s=w1146, f=w1160) -> (s? t:f=w1141:u64)
                        n472 = Greater?(x=w1159, y=w1141) -> (0:w1140:bool)
                        n473 = Select(t=w1141, s=w1140, f=w1136) -> (s? t:f=w1157:u64)
                        n474 = feedback-in #40(w1157) -> ()
                        n475 = Equal?(x="Scan steps", y=w1141) -> (x = y?=w1145:bool)
                        n476 = Greater?(x="Scan steps", y=w1129) -> (0:w1156:bool)
                        n477 = feedback #41(w1137) -> (w1158:i64)
                        n478 = Select(t=w1137, s=w1153, f=w1158) -> (s? t:f=w1143:i64)
                        n479 = Increment(x=w1143) -> (x+1=w1155:i64)
                        n480 = Decrement(x=w1143) -> (x-1=w1154:i64)
                        n481 = Select(t=w1155, s=w1156, f=w1154) -> (s? t:f=w1144:i64)
                        n482 = Select(t=w1143, s=w1145, f=w1144) -> (s? t:f=w1142:i64)
                        n483 = Select(t=w1143, s=w1146, f=w1142) -> (s? t:f=w1138:i64)
                        n484 = Select(t=w1138, s=w1140, f=w1137) -> (s? t:f=w1139:i64)
                        n485 = feedback-in #41(w1139) -> ()
                        n486 = feedback #42(w1136) -> (w1152:u64)
                        n487 = Select(t=w1136, s=w1153, f=w1152) -> (s? t:f=w1148:u64)
                        n488 = Increment(x=w1148) -> (x+1=w1149:u64)
                        n489 = Select(t=w1148, s=w1140, f=w1149) -> (s? t:f=w1147:u64)
                        n490 = Greater?(x="Number of scans", y=w1147) -> (0:w1133:bool)
                        n491 = Multiply(x="Scan freq.  increment", y=w1143) -> (x*y=w1128:i64)
                        n492 = Select(t=TRUE, s="Cont. Scan", f=w1133) -> (s? t:f=w1130:bool)
                        n493 = Select(t=w1147, s=w1130, f=w1136) -> (s? t:f=w1150:u64)
                        n494 = feedback-in #42(w1150) -> ()
                        n495 = local read "BD 1 Frequency 1"() -> (w1127:u64)
                        n496 = Increment(x=w1147) -> (x+1=→"Scan I":u64)
                        n497 = Add(x=w1128, y=w1127) -> (x+y=w1126:u64)
                        "Actual Scan freq" <- w1126
                      }
                      frame True {
                        n498 = local read "Actual Scan freq"() -> (w1164:u64)
                        n499 = local read "Scan steps"() -> (w1165:u64)
                      }
                    }
                    "Scanning" <- w1110
                    n500 = case shown="True" w1102 {
                      tunnel: w1105 -> [_ w1125]
                      frame False {
                      }
                      frame True {
                        n501 = Add(x=w1125, y=i16 2) -> (x+y=w1123:u64)
                        n502 = local write "Raster to target force"(FALSE) -> ()
                        n503 = local write "Scan steps"(w1123) -> ()
                      }
                    }
                  }
                }
                n504 = feedback #43(fxp<+/-,24,9> 0.0 ("AI1 X Set 2")) -> (w1085:fxp<+/-,24,9>)
                n505 = Select(t=w1073, s=w1047, f=w1085) -> (s? t:f=w1086:fxp<+/-,24,9>)
                "Trap Pos FB Int Signal" <- w1086
                n506 = feedback-in #43(w1086) -> ()
                n507 = feedback #44(fxp<+/-,16,1> 0.0 ("Trap Pos FB Int-Norm Signal")) -> (w1070:fxp<+/-,16,1>)
                n508 = Select(t=w1044, s=w1047, f=w1070) -> (s? t:f=w1069:fxp<+/-,16,1>)
                "Trap Pos FB Int-Norm Signal" <- w1069
                n509 = feedback-in #44(w1069) -> ()
                n510 = case "For position feedback" shown="True" "Force feedback" {
                  tunnel: [i64 0 w1197] -> w1054
                  tunnel: w1044 -> [_ w1194]
                  tunnel: w1047 -> [_ w1193]
                  frame False {
                  }
                  frame True {
                    n511 = feedback #45(i64 0) -> (w1196:i64)
                    n512 = case shown="True" w1193 {
                      tunnel: [w1198 w1202] -> w1197
                      tunnel: w1196 -> [w1198 _]
                      tunnel: w1194 -> [_ w1201]
                      frame False {
                      }
                      frame True {
                        n513 = xnode ("PID")("process variable"=w1201, "reset?"="Trap Pos. FB Reset", "setpoint"="Trap Pos. FB SP", "PID gains"="Trap Pos. FB Gains", "output range"="Trap pos. FB Range") -> ("output"=w1211:fxp<+/-,16,1>)
                        n514 = Negate(x=w1211) -> (-x=w1210:fxp<+/-,17,2>)
                        n515 = Select(t=w1210, s="Trap Pos FB Negate Action", f=w1211) -> (s? t:f=w1207:fxp<+/-,17,2>)
                        n516 = Scale By Power Of 2(n=u32 15, x=u32 1) -> (x*2^n=w1204:u32)
                        n517 = Multiply(x=w1207, y=w1204) -> (x*y=w1203:fxp<+/-,17,17>)
                        n518 = To Quad Integer(1:w1203) -> (0:w1215:i64)
                        "Trap Pos FB Action" <- w1215
                        n519 = Multiply(x=w1215, y="Trap Pos. FB Mult Factor") -> (x*y=w1213:i64)
                        n520 = Add(x=w1213, y="Trap Pos. FB Offset Factor") -> (x+y=w1202:i64)
                        n521 = disable-structure shown="Disabled" {
                          disable-tunnel: w1202 -> [w1222 _]
                          frame Disabled {
                            w1226 = u32 0
                            n522 = feedback #46() -> (w1223:i64)  [unwired: 1 in]
                            n523 = Add(x=w1222, y=w1223) -> (x+y=w1220:i64)
                            n524 = feedback #47(w1226) -> (w1228:u32)
                            n525 = Increment(x=w1228) -> (x+1=w1217:u32)
                            n526 = Greater Or Equal?(x=w1217, y="FB Trig Integrate") -> (x >= y?=w1218:bool)
                            n527 = Select(t=i64 0, s=w1218, f=w1220) -> (s? t:f=w1224:i64)
                            n528 = feedback-in #46(w1224) -> ()
                            n529 = Select(t=w1226, s=w1218, f=w1217) -> (s? t:f=w1227:u32)
                            n530 = feedback-in #47(w1227) -> ()
                            n531 = And(x=w1218, y="FPGA Trap Trig") -> (x .and. y?=w1225:bool)
                            n532 = case "Trap FB trigger excitation laser ON" shown="True" w1225 {
                              tunnel: w1220 -> [_ w1232]
                              tunnel: w1217 -> [_ w1230]
                              frame False {
                              }
                              frame True {
                                n533 = Not(x="TTrig Negate Pos") -> (.not. x?=w1239:bool)
                                n534 = Boolean To (0,1)(Boolean="TTrig Negate Pos") -> (0, 1=w1237:i16)
                                n535 = Boolean To (0,1)(Boolean=w1239) -> (0, 1=w1238:i16)
                                n536 = Negate(x=w1237) -> (-x=w1236:i16)
                                n537 = Add(x=w1236, y=w1238) -> (x+y=w1235:i16)
                                n538 = Multiply(x=w1235, y=w1232) -> (x*y=w1234:i64)
                                "TTrig Sig" <- w1234
                                n539 = Multiply(x="FPGA TTrig Thresh", y=w1230) -> (x*y=w1231:i64)
                                "TTrig Fin Thresh" <- w1231
                                n540 = Greater Or Equal?(x=w1234, y=w1231) -> (x >= y?=w1233:bool)
                                n541 = case shown="True" w1233 {
                                frame False {
                                }
                                frame True {
                                w1242 = TRUE ("Green FB On/Off")
                                w1244 = u8 2 ("Operating Mode")
                                n542 = local write "Operating Mode"(w1244) -> ()
                                n543 = local write item#-1(w1244) -> ()
                                n544 = local write item#-1(w1242) -> ()
                                n545 = local write "FPGA Trap Trig"(FALSE ("FPGA Trap Trig")) -> ()
                                "TTrig?" <- w1242
                                }
                                }
                              }
                            }
                          }
                          frame Enabled {
                          }
                        }
                      }
                    }
                    n546 = feedback-in #45(w1197) -> ()
                  }
                }
                n547 = And(x="Force feedback", y="Dynamic Force FB (Ronen)") -> (x .and. y?=w1055:bool)
                n548 = case shown="True" w1055 {
                  tunnel: w1054 -> [w1169 w1173]
                  tunnel: [w1168 w1172] -> w1040
                  tunnel: w1048 -> [_ w1171]
                  tunnel: w1047 -> [_ w1170]
                  frame False {
                    # "(BD1 Frequency 1)"
                    n549 = Add(x="BD 1 Frequency 1", y=w1169) -> (x+y=w1168:u64)
                  }
                  frame True {
                    n550 = case shown="True" w1170 {
                      tunnel: w1173 -> [_ w1177]
                      tunnel: [w1174 w1176] -> w1172
                      tunnel: w1171 -> [w1174 w1175]
                      frame False {
                      }
                      frame True {
                        n551 = Add(x=w1175, y=w1177) -> (x+y=w1176:u64)
                      }
                    }
                  }
                }
                n552 = case shown="True" w1038 {
                  tunnel: [w1094 w1096] -> w1041
                  tunnel: w1040 -> [w1094 _]
                  tunnel: w1039 -> [_ w1096]
                  frame False {
                  }
                  frame True {
                    n553 = local write "BD 1 Frequency 1"(w1096) -> ()
                    n554 = local write "Abort scan"(FALSE) -> ()
                  }
                }
                n555 = Select(t=w1065, s="Trap 1 osc enable", f=i64 0) -> (s? t:f=w1063:i64)
                n556 = Select(t=w1088, s="Scan BD", f=w1045) -> (s? t:f=w1087:u64)
                n557 = Select(t=w1045, s="Scan BD", f=w1088) -> (s? t:f=w1053:u64)
                n558 = Add(x=w1087, y=w1062) -> (x+y=w1090:u64)
                n559 = Compound Arithmetic op=ADD(w1063, w1041, w1053) -> (w1052:u64)
                n560 = In Range and Coerce(upper limit="FB Max Frequency", x=w1052, lower limit="FB Min frequency") -> (coerced(x)=w1049:u64)  [unwired: 1 out]
                "BD1 Frequency Out 1" <- w1049
              }
              frame 2 {
                # "Trap 2"
                n561 = case "Trap 2 X intensity feedback" shown="True" "FB On/Off Set 2" {
                  tunnel: [w1295 w1298] -> w1281
                  tunnel: "BD 1 Amplitude 2" -> [w1295 _]
                  tunnel: w1291 -> [_ w1297]
                  tunnel: w1290 -> [_ w1296]
                  frame False {
                  }
                  frame True {
                    n562 = local read "AI2 Y Sum Set 2"() -> (w1301:i16)
                    n563 = call "Slower PID.vi"("process variable"=w1301, "reset?"="FB Reset Set 2", "setpoint"="FB Setpoint Set 2", "PID gains (x 2^8)"=w1297, "output range"=w1296) -> ("output"=w1299:i16)  [unwired: 10 out]
                    n564 = To Unsigned Word Integer(number=w1299) -> (unsigned 16bit integer=w1298:u16)
                  }
                }
                "BD1 amplitude 2 out" <- w1281
                n565 = Select(t=w1288, s="Trap 2 osc enable", f=i64 0) -> (s? t:f=w1287:i64)
                n566 = Add(x="BD 1 Frequency 2", y=w1287) -> (x+y=w1285:u64)
                "BD1 Frequency Out 2" <- w1285
              }
              frame 3 {
                # "Fluorescence period"
                n567 = disable-structure shown="Disabled" {
                  disable-tunnel: [w1314 _] -> w1305
                  disable-tunnel: w1304 -> [w1313 _]
                  frame Disabled {
                    # "Remember if FB was previously on/off"
                    n568 = feedback #48(FALSE) -> (w1309:bool)
                    n569 = case shown="True" w1313 {
                      tunnel: [w1316 w1332] -> w1314
                      tunnel: "BD 2 Amplitude 3" -> [w1316 _]
                      tunnel: [FALSE TRUE] -> w1310
                      tunnel: w1309 -> [_ w1318]
                      frame False {
                      }
                      frame True {
                        # "Makes it so first time FB run when turned on, the PID sees the detector intensity from the last time FB was running, rather than something near zero. Especially assuming the setpoint is not changing, this will make the FB more stable when resuming, and not overshoot the turnon intensity."
                        # "FB output range: 0 should be low, full scale is 12 bits.\nBut be careful not to go over, then higher bits just get ignored by RF board, so output will actually jump down and be unstable. Keep it under 4000 to be safe."
                        n570 = local read "Green FB Sum"() -> (w1317:i16)
                        n571 = feedback-in #49(w1317) -> ()
                        n572 = feedback #49(i16 0 ("Green FB Sum")) -> (w1320:i16)
                        n573 = Select(t=w1317, s=w1318, f=w1320) -> (s? t:f=w1319:i16)
                        n574 = Bundle("P3 2"="P3 2", "I3 2"="I3 2", "D3 2"="D3 2") -> (w1331:cluster{"P3 2":i16, "I3 2":i16, "D3 2":i16})  [unwired: 1 in]
                        n575 = Bundle("RF synth green feedback max"="RF synth green feedback max", i16 0) -> (w1323:cluster{"RF synth green feedback max":i16, i16})  [unwired: 1 in]
                        n576 = call "Slower PID.vi"("process variable"=w1319, "reset?"="Green FB Reset 2", "setpoint"="Green FB Setpoint 2", "PID gains (x 2^8)"=w1331, "output range"=w1323) -> ("output"=w1333:i16)  [unwired: 10 out]
                        n577 = To Unsigned Word Integer(number=w1333) -> (unsigned 16bit integer=w1332:u16)
                      }
                    }
                    n578 = feedback-in #48(w1310) -> ()
                  }
                  frame Enabled {
                  }
                }
              }
            }
            n579 = Split Number(x=w874) -> (hi(x)=w873:u32, lo(x)=w872:u32)
            n580 = Boolean To (0,1)(Boolean="+ phase (DIO)") -> (0, 1=w834:i16)
            n581 = Split Number(x=w873) -> (lo(x)=w871:u16)  [unwired: 1 out]
            n582 = Split Number(x=w872) -> (hi(x)=w870:u16, lo(x)=w869:u16)
            n583 = Split Number(x=w871) -> (hi(x)=w863:u8, lo(x)=w862:u8)
            n584 = Split Number(x=w870) -> (hi(x)=w861:u8, lo(x)=w860:u8)
            n585 = Split Number(x=w869) -> (hi(x)=w859:u8, lo(x)=w858:u8)
            n586 = Multiply(x=w834, y="Phase count adjustment (DIO)") -> (x*y=w830:i16)
            n587 = feedback #50(TRUE) -> (w819:bool)
            n588 = Not(x=w819) -> (.not. x?=w818:bool)
            n589 = feedback-in #50(w818) -> ()
            n590 = feedback #51(i16 0) -> (w832:i16)
            n591 = Subtract(x=w832, y=w830) -> (x-y=w831:i16)
            "DIO Relative phase" <- w831
            n592 = feedback-in #51(w831) -> ()
            n593 = Add(x=w837, y=w830) -> (x+y=w836:u32)
            n594 = Build Array "BD 1 nu Stack"(w863, w862, w861, w860, w859, w858) -> (w857:u8[])
            n595 = Not Equal?(x=w797, y=u8 3) -> (x != y?=w806:bool)
            n596 = case "Store in RF board F1 or F2" shown="True" w818 {
              tunnel: [w1029 w1033] -> w848
              tunnel: [u8 10 u8 4] -> w849
              tunnel: "Swap F1 and F2" -> [w1030 w1033]
              tunnel: "BD 2 Frequency 1" -> [_ w1032]
              tunnel: "BD 2 Frequency 2" -> [w1028 _]
              tunnel: [w1028 w1032] -> w814
              frame False {
                # "for RF synth controls\ngreen: F1/F2 stay same"
                # "F2 address (hex)"
                n597 = Not(x=w1030) -> (.not. x?=w1029:bool)
              }
              frame True {
                # "low chooses F1"
                # "F1 address (hex)"
              }
            }
            n598 = Select(t=w814, s="RF synth bd controls green", f=w813) -> (s? t:f=w812:u64)
            n599 = Split Number(x=w812) -> (hi(x)=w868:u32, lo(x)=w867:u32)
            n600 = Split Number(x=w868) -> (lo(x)=w866:u16)  [unwired: 1 out]
            n601 = Split Number(x=w867) -> (hi(x)=w865:u16, lo(x)=w864:u16)
            n602 = Split Number(x=w866) -> (hi(x)=w856:u8, lo(x)=w855:u8)
            n603 = Split Number(x=w865) -> (hi(x)=w854:u8, lo(x)=w853:u8)
            n604 = Split Number(x=w864) -> (hi(x)=w852:u8, lo(x)=w851:u8)
            n605 = feedback #52(u16 0 ("BD 2 Amplitude 3")) -> (w803:u16)
            n606 = Select(t=w803, s=w806, f=w805) -> (s? t:f=w804:u16)
            n607 = feedback-in #52(w804) -> ()
            n608 = And(x=w806, y=w809) -> (x .and. y?=w808:bool)
            n609 = Build Array "BD 2 nu Stack"(w856, w855, w854, w853, w852, w851) -> (w850:u8[])
            n610 = Select(t=w803, s=w808, f=w805) -> (s? t:f=w786:u16)
            n611 = flat-sequence "Update trap RF synth board settings to be used for the upcoming trap cycle." {
              tunnel: w850 -> [w977]
              tunnel: w857 -> [w978]
              tunnel: [w978] -> w801
              tunnel: [w977] -> w800
              tunnel: w849 -> [w979]
              tunnel: w801 -> [w981]
              tunnel: w800 -> [w980]
              tunnel: w788 -> [w992]
              tunnel: w790 -> [w991]
              tunnel: w789 -> [w990]
              frame #0 {
                # "To possibly delay\nthese writes to very\nend of loop (for x and\ny phase adjust)"
                n612 = call "Wait8"("Count(Ticks)"="Next trap write delay (ticks)") -> ()  [unwired: 1 out]
              }
              frame #1 {
                # "Next trap RF frequency:\n\nWrite next trap cycle frequency to buffer."
                n613 = for {
                  tunnel: w981 -> [w987] mode=indexing
                  tunnel: w980 -> [w986] mode=indexing
                  tunnel: w979 -> [w984]
                  i -> [w985]
                  n614 = To Unsigned Byte Integer(number=w985) -> (unsigned 8bit integer=w982:u8)
                  n615 = Add(x=w984, y=w982) -> (x+y=w983:u8)
                  n616 = call "write to RF synth bd.vi"("Address Byte"=w983, "BD 2 Byte"=w986, "BD 1 Byte"=w987) -> ()
                }
              }
              frame #2 {
                w988 = TRUE ("Connector1/DIO15")
                # "Send udclk high\n(BD 1 and 2) to make the new frequency active in F1 or F2 word. But it won't actually be the used frequency until FSK switches to it (begining of next cycle)."
                n617 = xnode "FPGA I/O Node"("Connector1/DIO30"=w988, "Connector1/DIO29"=w988) -> ()  [unwired: 2 in, 2 out]
              }
              frame #3 {
                w989 = FALSE ("Connector1/DIO15")
                n618 = xnode "FPGA I/O Node"("Connector1/DIO30"=w989, "Connector1/DIO29"=w989) -> ()  [unwired: 2 in, 2 out]
              }
              frame #4 {
                # "Next trap RF phase offset:\n\nSet the next trap cycle amplitude to the buffer. Won't become active until udclk is set high at proper time at the begining of the next cycle."
                n619 = case shown="True" w992 {
                  tunnel: w991 -> [_ w993]
                  tunnel: w990 -> [_ w994]
                  frame False {
                  }
                  frame True {
                    # "phase 1 address start"
                    n620 = for {
                      tunnel: w993 -> [w1001] mode=indexing
                      tunnel: w994 -> [w1000] mode=indexing
                      tunnel: u8 0 -> [w998]
                      i -> [w999]
                      n621 = To Unsigned Byte Integer(number=w999) -> (unsigned 8bit integer=w996:u8)
                      n622 = Add(x=w998, y=w996) -> (x+y=w997:u8)
                      n623 = call "write to RF synth bd.vi"("Address Byte"=w997, "BD 2 Byte"=w1000, "BD 1 Byte"=w1001) -> ()
                    }
                  }
                }
              }
              frame #5 {
                # "Prep to reset RF phase to zero at start of next cycle. Only reset BD 1. Do nothing to BD 2. This puts the settings in the buffer. A udclk high will make both this phase reset and possibly a new phase offset setting active."
                n624 = case shown="True" "RF phase reset before cycles" {
                  frame False {
                  }
                  frame True {
                    w1004 = u8 66  # BD 1 reset
                    n625 = call "write to RF synth bd.vi"("Address Byte"=u8 31, "BD 2 Byte"=u8 2, "BD 1 Byte"=w1004) -> ()
                  }
                }
              }
              frame #6 {
                # "Address"
                # "Data BD 2"
                # "Data BD 1"
                # "If phase reset wasn't chosen previously, these actions will have no affect. For both BD's, data should be binary 10, and address should be hex 1F (bin 01 1111)"
                # "This sets up the digital communication lines to restart phase accumulation (start RF running agin). It cancels out the possible phase reset. Just need to set WR DIO low then udclk DIOhigh  to make this happen. Doing this here early (and not using the usual board write function) speeds things up.\n\nRestarts RF (BD 1 only, BD2 never stopped in first place)."
                n626 = xnode "FPGA I/O Node"("Connector1/DIO0"=FALSE, "Connector1/DIO1"=FALSE, "Connector1/DIO2"=FALSE, "Connector1/DIO3"=FALSE, "Connector1/DIO4"=FALSE, "Connector1/DIO5"=FALSE, "Connector1/DIO6"=TRUE, "Connector1/DIO7"=FALSE, "Connector1/DIO8"=FALSE, "Connector1/DIO9"=TRUE, "Connector1/DIO10"=TRUE, "Connector1/DIO11"=TRUE, "Connector1/DIO12"=TRUE, "Connector1/DIO13"=TRUE, "Connector1/DIO20"=FALSE, "Connector1/DIO21"=FALSE, "Connector1/DIO22"=FALSE, "Connector1/DIO23"=FALSE, "Connector1/DIO24"=FALSE, "Connector1/DIO25"=FALSE, "Connector1/DIO26"=TRUE, "Connector1/DIO27"=FALSE) -> ()  [unwired: 22 in, 22 out]
              }
            }
            n627 = feedback #53(fxp<+,8,8> 0.0) -> (w783:fxp<+,8,8>)
            n628 = Increment(x=w783) -> (x+1=w781:fxp<+,8,8>)
            n629 = feedback-in #53(w781) -> ()
            n630 = case "Trap RF phase offset control methods" shown="3" "Phase offset method" {
              tunnel: [fxp<+,14,14> 0.0 ("Phase BD 1") w927 w942 w971] -> w791
              tunnel: "Phase Trap 1" -> [_ w928 w943 _]
              tunnel: w797 -> [_ w929 w944 w972]
              tunnel: [FALSE TRUE TRUE TRUE] -> w788
              tunnel: "Phase Trap 2" -> [_ w925 w940 _]
              tunnel: w781 -> [_ _ w939 _]
              frame 0, Default {
              }
              frame 1 {
                # "Constant increment of phase offset with each trap cycle. This results in a constant phase difference between trap cycles. \nOnly for traps 1 and 2 (set phase offset to zero for set three)."
                n631 = case shown="1, Default" w929 {
                  tunnel: w928 -> [_ _ w935]
                  tunnel: [w931 fxp<+,14,14> 0.0 w936] -> w927
                  tunnel: w925 -> [w930 _ _]
                  frame 2 {
                    n632 = feedback #54(fxp<+,14,14> 0.0) -> (w933:fxp<+,14,14>)
                    n633 = Add(x=w930, y=w933) -> (x+y=w931:fxp<+,14,14>)
                    n634 = feedback-in #54(w931) -> ()
                  }
                  frame 3 {
                  }
                  frame 1, Default {
                    n635 = feedback #55(fxp<+,14,14> 0.0) -> (w938:fxp<+,14,14>)
                    n636 = Add(x=w935, y=w938) -> (x+y=w936:fxp<+,14,14>)
                    n637 = feedback-in #55(w936) -> ()
                  }
                }
              }
              frame 2 {
                # "Changing increment of phase offset with each trap cycle. This results in a constant change in phase difference between trap cycles. \nOnly for traps 1 and 2 (set phase offset to zero for set three)."
                n638 = case shown="2" w944 {
                  tunnel: w943 -> [_ _ w954]
                  tunnel: [w945 fxp<+,14,14> 0.0 w952] -> w942
                  tunnel: w940 -> [w947 _ _]
                  tunnel: w939 -> [w948 _ w955]
                  frame 2 {
                    n639 = Multiply(x=w947, y=w948) -> (x*y=w946:fxp<+,16,16>)
                    n640 = feedback #56(fxp<+,14,14> 0.0) -> (w950:fxp<+,14,14>)
                    n641 = Add(x=w946, y=w950) -> (x+y=w945:fxp<+,14,14>)
                    n642 = feedback-in #56(w945) -> ()
                  }
                  frame 3 {
                  }
                  frame 1, Default {
                    n643 = Multiply(x=w954, y=w955) -> (x*y=w953:fxp<+,16,16>)
                    n644 = feedback #57(fxp<+,14,14> 0.0) -> (w957:fxp<+,14,14>)
                    n645 = Add(x=w953, y=w957) -> (x+y=w952:fxp<+,14,14>)
                    n646 = feedback-in #57(w952) -> ()
                  }
                }
              }
              frame 3 {
                w964 = u32 1013904223  # LCG constant C (add)
                w966 = fxp<+,21,21> 1664525.0  # LCG constant A (multiply)
                # "Set a random phase offset. Random number generated using the LCG method. Constants and method taken from NI white noise generator code (method is general though)."
                # "shift to 14 significant bits"
                n647 = feedback #58(u32 4294967295 ("seed")) -> (w961:u32)
                n648 = Multiply(x=w961, y=w966) -> (x*y=w965:u32)
                n649 = Split Number(x=w961) -> (hi(x)=w967:u16)  [unwired: 1 out]
                n650 = To Unsigned Word Integer(number=w967) -> (unsigned 16bit integer=w959:u16)
                n651 = Add(x=w965, y=w964) -> (x+y=w963:fxp<+,32,32>)
                n652 = To Unsigned Long Integer(number=w963) -> (unsigned 32bit integer=w960:u32)
                n653 = feedback-in #58(w960) -> ()
                n654 = Scale By Power Of 2(n=i8 -2 ("Uniform scale factor"), x=w959) -> (x*2^n=w968:u16)
                n655 = To Fixed-Point(number=w968) -> (fixed-point=w958:fxp<+,14,14>)  [unwired: 1 in]
                "Random phase generated" <- w958
                n656 = case shown="1, Default" w972 {
                  tunnel: [w973 fxp<+,14,14> 0.0 w975] -> w971
                  tunnel: w958 -> [w973 _ w975]
                  frame 2 {
                  }
                  frame 3 {
                  }
                  frame 1, Default {
                  }
                }
              }
            }
            n657 = To Unsigned Word Integer(number=w791) -> (unsigned 16bit integer=w796:u16)
            n658 = Split Number(x=w796) -> (hi(x)=w794:u8, lo(x)=w795:u8)
            n659 = Split Number(x=u16 0) -> (hi(x)=w792:u8, lo(x)=w793:u8)
            n660 = Build Array ("BD 1 A Stack")(w794, w795) -> (w790:u8[])
            n661 = Build Array ("BD 1 A Stack")(w792, w793) -> (w789:u8[])
          }
        }
      }
    }
  }
  n662 = while "532 nm green fluorescent laser interlacing (DO to IA 532 nm AOM ME amp)." {
    shift-right: [w1337] -> _
    shift-left: w6 -> [w1342]
    shift-right: [w1336] -> _
    shift-left: w7 -> [w1334]
    stop <- FALSE stop-if-true
    n663 = flat-sequence {
      tunnel: w1342 -> [w1345]
      tunnel: [w1344] -> w1340
      tunnel: [w1345] -> w1338
      tunnel: [w1346] -> w1335
      tunnel: w1334 -> [w1346]
      tunnel: [w1349] -> w1341
      tunnel: w1340 -> [w1349]
      tunnel: [w1348] -> w1339
      tunnel: w1338 -> [w1348]
      tunnel: w1335 -> [w1347]
      tunnel: [w1361] -> w1337
      tunnel: w1341 -> [w1380]
      tunnel: w1339 -> [w1377]
      tunnel: [w1350] -> w1336
      frame #0 {
        n664 = call "Loop Timer9"("Count(Ticks)"=w1345) -> ("Tick Count(Ticks)"=w1344:u32)
      }
      frame #1 {
        # "Then to PRL 440 amp\nOR to RF synth board FSK in"
        n665 = xnode "FPGA I/O Node"("Connector1/DIO37"=w1347, "Connector1/DIO38"=w1347, "Connector1/DIO39"=w1347, "Connector1/DIO26"=w1347, "Connector1/DIO27"=w1347, "Connector1/DIO32"=w1347) -> ()  [unwired: 6 in, 6 out]
      }
      frame #2 {
        n666 = feedback-in #59(w1380) -> ()
        n667 = feedback #59(w1380) -> (w1379:u32)
        n668 = Subtract(x=w1380, y=w1379) -> (x-y=w1378:u32)
        n669 = Subtract(x=w1378, y=w1377) -> (x-y=w1354:u32)
        n670 = Number To Boolean Array(number=w1354) -> (Boolean array=w1355:bool[])
        n671 = Or Array Elements(Boolean array=w1355) -> (logical OR=w1353:bool)
        n672 = Boolean To (0,1)(Boolean="+ phase (GI)") -> (0, 1=w1366:i16)
        n673 = Boolean To (0,1)(Boolean=w1353) -> (0, 1=w1360:i16)
        n674 = To Unsigned Byte Integer(number=w1360) -> (unsigned 8bit integer=w1357:u8)
        n675 = Multiply(x=w1366, y="Phase count adjustment (GI)") -> (x*y=w1363:i16)
        n676 = feedback #60(u8 0) -> (w1358:u8)
        n677 = Add(x=w1357, y=w1358) -> (x+y=w1356:u8)
        "GI Late Counter" <- w1356
        n678 = feedback-in #60(w1356) -> ()
        n679 = feedback #61(i16 0) -> (w1364:i16)
        n680 = Subtract(x=w1364, y=w1363) -> (x-y=w1362:i16)
        "GI Relative phase" <- w1362
        n681 = feedback-in #61(w1362) -> ()
        n682 = feedback #62(TRUE) -> (w1372:bool)
        n683 = case shown="2" "Operating Mode" {
          tunnel: [TRUE FALSE w1405] -> w1351
          tunnel: w1372 -> [_ _ w1402]
          frame 0, Default {
          }
          frame 1 {
          }
          frame 2 {
            n684 = Not(x=w1402) -> (.not. x?=w1404:bool)
            n685 = Select(t=w1404, s="Invert GI", f=w1402) -> (s? t:f=w1405:bool)
          }
        }
        n686 = Not(x=w1372) -> (.not. x?=w1369:bool)
        n687 = Select(t="Green interlace ON count", s=w1369, f="Green interlace OFF count") -> (s? t:f=w1374:u16)
        n688 = Subtract(x=w1374, y=w1354) -> (x-y=w1367:u32)
        n689 = Add(x=w1367, y=w1363) -> (x+y=w1361:u32)
        n690 = feedback-in #62(w1369) -> ()
        n691 = case shown="True" "Green long-scale interlacing" {
          tunnel: w1351 -> [w1381 w1389]
          tunnel: [w1381 w1390] -> w1350
          frame False {
          }
          frame True {
            n692 = feedback #63(i16 1) -> (w1396:i16)
            n693 = Increment(x=w1396) -> (x+1=w1395:i16)
            n694 = feedback #64("Number of ON cycles") -> (w1382:i16)
            n695 = Greater?(x=w1382, y=w1396) -> (0:w1391:bool)
            n696 = Select(t=w1395, s=w1391, f=i16 1) -> (s? t:f=w1393:i16)
            n697 = feedback-in #63(w1393) -> ()
            n698 = feedback #65(TRUE) -> (w1388:bool)
            n699 = Not(x=w1388) -> (.not. x?=w1387:bool)
            n700 = Select(t=w1388, s=w1391, f=w1387) -> (s? t:f=w1386:bool)
            n701 = Select(t="Number of ON cycles", s=w1386, f="Number of OFF cycles") -> (s? t:f=w1384:i16)
            n702 = feedback-in #64(w1384) -> ()
            n703 = feedback-in #65(w1386) -> ()
            n704 = case shown="False" w1386 {
              tunnel: [FALSE w1399] -> w1390
              tunnel: w1389 -> [_ w1399]
              frame False {
              }
              frame True {
              }
            }
          }
        }
      }
    }
  }
  n705 = while "Green excitation laser feedback measurement" {
    shift-right: [w1406] -> _
    shift-left: w6 -> [w1411]
    stop <- FALSE stop-if-true
    n706 = flat-sequence {
      tunnel: w1411 -> [w1413]
      tunnel: [w1414] -> w1409
      tunnel: [w1413] -> w1407
      tunnel: [w1421] -> w1410
      tunnel: w1409 -> [w1421]
      tunnel: [w1420] -> w1408
      tunnel: w1407 -> [w1420]
      tunnel: [w1433] -> w1406
      tunnel: w1410 -> [w1444]
      tunnel: w1408 -> [w1441]
      frame #0 {
        n707 = call "Loop Timer6"("Count(Ticks)"=w1413) -> ("Tick Count(Ticks)"=w1414:u32)
      }
      frame #1 {
        n708 = xnode "FPGA I/O Node"("Connector1/DIO35"=TRUE) -> ("Chassis2/Mod2/AI0"=w1419:i16, "Chassis2/Mod2/AI1"=w1418:i16, "Chassis2/Mod2/AI2"=w1415:i16)  [unwired: 4 in, 4 out]
        "Green FB Sum" <- w1415
        n709 = Bundle("Chassis2/Mod2/AI0"=w1419, "Chassis2/Mod2/AI1"=w1418, "Chassis2/Mod2/AI2"=w1415) -> (→"Green FB Signals":T10)  [unwired: 1 out]
      }
      frame #2 {
        n710 = feedback-in #66(w1444) -> ()
        n711 = feedback #66(w1444) -> (w1443:u32)
        n712 = Subtract(x=w1444, y=w1443) -> (x-y=w1442:u32)
        n713 = xnode "FPGA I/O Node"("Connector1/DIO35"=FALSE) -> ()  [unwired: 1 in, 1 out]
        n714 = Subtract(x=w1442, y=w1441) -> (x-y=w1423:u32)
        n715 = Subtract(x="Green FB Count", y=w1423) -> (x-y=w1437:u32)
        n716 = Number To Boolean Array(number=w1423) -> (Boolean array=w1424:bool[])
        n717 = Or Array Elements(Boolean array=w1424) -> (logical OR=w1422:bool)
        "Green FB Late?" <- w1422
        n718 = Boolean To (0,1)(Boolean="+ phase (Green FB)") -> (0, 1=w1435:i16)
        n719 = Boolean To (0,1)(Boolean=w1422) -> (0, 1=w1429:i16)
        n720 = Multiply(x=w1435, y="Phase count adjustment (Green FB)") -> (x*y=w1430:i16)
        n721 = Add(x=w1437, y=w1430) -> (x+y=w1433:u32)
        n722 = To Unsigned Word Integer(number=w1429) -> (unsigned 16bit integer=w1426:u16)
        n723 = feedback #67(i16 0) -> (w1432:i16)
        n724 = Subtract(x=w1432, y=w1430) -> (x-y=w1431:i16)
        "Green FB Relative Phase" <- w1431
        n725 = feedback-in #67(w1431) -> ()
        n726 = feedback #68(u16 0) -> (w1427:u16)
        n727 = Add(x=w1426, y=w1427) -> (x+y=w1425:u16)
        "Green Late Counter" <- w1425
        n728 = feedback-in #68(w1425) -> ()
      }
    }
  }
  n729 = while "Control APD data integration - stream to host" {
    shift-right: [w1447] -> _
    shift-left: w9 -> [w1452]
    stop <- FALSE stop-if-true
    n730 = flat-sequence {
      tunnel: w1452 -> [w1454]
      tunnel: [w1455] -> w1450
      tunnel: [w1454] -> w1448
      tunnel: [w1467] -> w1451
      tunnel: w1450 -> [w1467]
      tunnel: [w1466] -> w1449
      tunnel: w1448 -> [w1466]
      tunnel: [w1464] -> w1446
      tunnel: [w1463] -> w1445
      tunnel: [w1503] -> w1447
      tunnel: w1451 -> [w1514]
      tunnel: w1449 -> [w1511]
      tunnel: w1446 -> [w1496]
      tunnel: w1445 -> [w1495]
      frame #0 {
        n731 = call "Loop Timer4"("Count(Ticks)"=w1454) -> ("Tick Count(Ticks)"=w1455:u32)
      }
      frame #1 {
        w1457 = 0 ("Timeout")
        n732 = node-c288() -> (w1462:T7)  [unwired: 1 in]
        n733 = timed-loop {
          timing: w1462 -> [_]
          timing-out: [_] -> w1461
          tunnel: [w1472] -> w1464
          tunnel: [w1471] -> w1463
          tunnel: [w1469] -> w1456
          tunnel: [w1468] -> w1460
          stop <- TRUE stop-if-true
          n734 = xnode ("FIFO Write")() -> ("Number of Elements to Read"=w1472:u32, "FIFO Out"=w1469:refnum<k21>)  [unwired: 1 in]
          n735 = xnode ("FIFO Write")() -> ("Number of Elements to Read"=w1471:u32, "FIFO Out"=w1468:refnum<k21>)  [unwired: 1 in]
        }
        n736 = case shown="True" "APD to FIFO" {
          tunnel: w1464 -> [_ w1479]
          tunnel: w1463 -> [_ w1477]
          frame False {
          }
          frame True {
            n737 = flat-sequence {
              tunnel: 0 ("Timeout") -> [w1481]
              tunnel: w1479 -> [w1482]
              tunnel: [w1481] -> w1478
              tunnel: w1478 -> [w1484]
              tunnel: w1477 -> [w1483]
              frame #0 {
                n738 = xnode ("FIFO Write")("Element"=w1482, "Timeout"=w1481) -> ()  [unwired: 1 in, 2 out]
              }
              frame #1 {
                n739 = xnode ("FIFO Write")("Element"=w1483, "Timeout"=w1484) -> ()  [unwired: 1 in, 2 out]
              }
            }
          }
        }
        n740 = node-c288(w1461) -> ()
        n741 = xnode "FIFO Read"("Timeout"=w1457, "FIFO In"=w1456) -> ("FIFO Out"=w1459:refnum<k21>)  [unwired: 2 out]
        n742 = xnode "FIFO Read"("Timeout"=w1457, "FIFO In"=w1460) -> ("FIFO Out"=w1458:refnum<k21>)  [unwired: 2 out]
        n743 = xnode ("FIFO Write")("FIFO In"=w1458) -> ()  [unwired: 1 out]
        n744 = xnode ("FIFO Write")("FIFO In"=w1459) -> ()  [unwired: 1 out]
      }
      frame #2 {
        n745 = feedback-in #69(w1514) -> ()
        n746 = feedback #69(w1514) -> (w1513:u32)
        n747 = Subtract(x=w1514, y=w1513) -> (x-y=w1512:u32)
        n748 = Subtract(x=w1512, y=w1511) -> (x-y=w1488:u32)
        n749 = Subtract(x="APD Acq Rate Count", y=w1488) -> (x-y=w1504:u32)
        n750 = Number To Boolean Array(number=w1488) -> (Boolean array=w1489:bool[])
        n751 = Or Array Elements(Boolean array=w1489) -> (logical OR=w1487:bool)
        "APD Acq Late?" <- w1487
        n752 = Boolean To (0,1)(Boolean=w1487) -> (0, 1=w1494:i16)
        n753 = To Unsigned Word Integer(number=w1494) -> (unsigned 16bit integer=w1491:u16)
        n754 = Boolean To (0,1)(Boolean="+ phase (APD Acq)") -> (0, 1=w1500:i16)
        n755 = feedback #70(u16 0) -> (w1492:u16)
        n756 = Add(x=w1491, y=w1492) -> (x+y=w1490:u16)
        "APD Acq Late Counter" <- w1490
        n757 = feedback-in #70(w1490) -> ()
        n758 = Multiply(x=w1500, y="Phase Count Adjustment (APD Acq)") -> (x*y=w1497:i16)
        n759 = Add(x=w1504, y=w1497) -> (x+y=w1503:u32)
        n760 = feedback #71(i16 0) -> (w1502:i16)
        n761 = Subtract(x=w1502, y=w1497) -> (x-y=w1499:i16)
        "APD Acq Relative Phase" <- w1499
        n762 = feedback-in #71(w1499) -> ()
        n763 = To Word Integer(number=w1496) -> (16bit integer=w1505:i16)
        n764 = To Word Integer(number=w1495) -> (16bit integer=w1506:i16)
        n765 = Multiply(x="APD 1 AO scale factor", y=w1505) -> (x*y=w1486:i16)
        n766 = Multiply(x="APD 2 AO scale factor", y=w1506) -> (x*y=w1485:i16)
        n767 = xnode "FPGA I/O Node"("Connector0/AO6"=w1486, "Connector0/AO7"=w1485) -> ()  [unwired: 2 in, 2 out]
      }
    }
  }
  n768 = node-c288(w3) -> ()
  n769 = node-c288(w1) -> ()
  n770 = disable-structure shown="Disabled" {
    disable-tunnel: w6 -> [w1515 _]
    frame Disabled {
      n771 = while "APD 3 Counter" {
        tunnel: w1515 -> [_]
        stop <- FALSE stop-if-true
        n772 = flat-sequence {
          frame #0 {
            n773 = xnode "FPGA I/O Method Node"("FPGA I/O In"=refnum<k21> "Connector0/DIO12" ("APD 2 DO"), "Timeout"=-1) -> ()  [unwired: 2 out]
          }
          frame #1 {
            n774 = local read "APD3 int gate"() -> (w1519:bool)
            n775 = case shown="True" w1519 {
              frame False {
              }
              frame True {
                n776 = local read item#-1() -> (w1520)
                n777 = case shown="True" w1520 {
                  frame False {
                    n778 = local read "APD 3 Counts 0"() -> (w1522:u32)
                    n779 = Increment(x=w1522) -> (x+1=→"APD 3 Counts 0":u32)
                  }
                  frame True {
                    n780 = local read "APD 3 Counts 1"() -> (w1524:u32)
                    n781 = Increment(x=w1524) -> (x+1=→"APD 3 Counts 1":u32)
                  }
                }
              }
            }
          }
        }
      }
    }
    frame Enabled {
    }
  }
  n782 = disable-structure shown="Disabled" {
    disable-tunnel: w6 -> [w1526 _]
    disable-tunnel: w8 -> [w1525 _]
    frame Disabled {
      n783 = while "APD 3 Gating" {
        shift-right: [w1530] -> _
        shift-left: w1526 -> [w1535]
        shift-right: [w1529] -> _
        shift-left: w1525 -> [w1527]
        stop <- FALSE stop-if-true
        n784 = flat-sequence {
          tunnel: w1535 -> [w1538]
          tunnel: [w1537] -> w1533
          tunnel: [w1538] -> w1531
          tunnel: [w1539] -> w1528
          tunnel: w1527 -> [w1539]
          tunnel: [w1542] -> w1534
          tunnel: w1533 -> [w1542]
          tunnel: [w1541] -> w1532
          tunnel: w1531 -> [w1541]
          tunnel: w1528 -> [w1540]
          tunnel: [w1563] -> w1530
          tunnel: w1534 -> [w1574]
          tunnel: w1532 -> [w1571]
          tunnel: [w1543] -> w1529
          frame #0 {
            n785 = call "Loop Timer5"("Count(Ticks)"=w1538) -> ("Tick Count(Ticks)"=w1537:u32)
          }
          frame #1 {
            # "Signal maybe then sent through \na transistor before APD"
            n786 = xnode "FPGA I/O Node"("Connector0/DIO2"=w1540) -> ()  [unwired: 1 in, 1 out]
            "APD3 int gate" <- w1540
          }
          frame #2 {
            n787 = local read "APD Gate OFF Count"() -> (w1548:u16)
            n788 = local read "APD Gate ON Count"() -> (w1549:u16)
            n789 = feedback #72(TRUE) -> (w1568:bool)
            n790 = feedback-in #73(w1574) -> ()
            n791 = feedback #73(w1574) -> (w1573:u32)
            n792 = Not(x=w1568) -> (.not. x?=w1566:bool)
            n793 = feedback-in #72(w1566) -> ()
            n794 = Subtract(x=w1574, y=w1573) -> (x-y=w1572:u32)
            n795 = Select(t=w1549, s=w1566, f=w1548) -> (s? t:f=w1570:u16)
            n796 = Subtract(x=w1572, y=w1571) -> (x-y=w1551:u32)
            n797 = Subtract(x=w1570, y=w1551) -> (x-y=w1562:u32)
            n798 = Number To Boolean Array(number=w1551) -> (Boolean array=w1552:bool[])
            n799 = Or Array Elements(Boolean array=w1552) -> (logical OR=w1550:bool)
            n800 = Boolean To (0,1)(Boolean=w1550) -> (0, 1=w1557:i16)
            n801 = Boolean To (0,1)(Boolean="+ phase (APD 3 Gate)") -> (0, 1=w1560:i16)
            n802 = To Unsigned Byte Integer(number=w1557) -> (unsigned 8bit integer=w1554:u8)
            n803 = Multiply(x=w1560, y="Phase count adjustment (APD 3 Gate)") -> (x*y=w1558:i16)
            n804 = feedback #74(u8 0) -> (w1555:u8)
            n805 = Add(x=w1554, y=w1555) -> (x+y=w1553:u8)
            "APD 3 Gate Late Counter" <- w1553
            n806 = feedback-in #74(w1553) -> ()
            n807 = Add(x=w1562, y=w1558) -> (x+y=w1563:u32)
            n808 = feedback #75(i16 0) -> (w1565:i16)
            n809 = Subtract(x=w1565, y=w1558) -> (x-y=w1564:i16)
            "APD 3 Gate Relative Phase" <- w1564
            n810 = feedback-in #75(w1564) -> ()
            n811 = local read "APD Gate Operating Mode"() -> (w1547:u8)
            n812 = case shown="2" w1547 {
              tunnel: [TRUE FALSE w1577] -> w1544
              tunnel: w1568 -> [_ _ w1577]
              frame 0, Default {
              }
              frame 1 {
              }
              frame 2 {
              }
            }
            n813 = local read "Invert APD Gate"() -> (w1546:bool)
            n814 = Not(x=w1544) -> (.not. x?=w1545:bool)
            n815 = Select(t=w1545, s=w1546, f=w1544) -> (s? t:f=w1543:bool)
          }
        }
      }
    }
    frame Enabled {
    }
  }
  n816 = disable-structure shown="Disabled" {
    disable-tunnel: w6 -> [w1580 _]
    disable-tunnel: w7 -> [w1579 _]
    frame Disabled {
      n817 = while "633 nm red  fluorescent laser interlacing (DO to IA 633 nm AOM ME amp)." {
        shift-right: [w1701] -> _
        shift-left: w1580 -> [w1706]
        shift-right: [w1700] -> _
        shift-left: w1579 -> [w1698]
        stop <- FALSE stop-if-true
        n818 = flat-sequence {
          tunnel: w1706 -> [w1709]
          tunnel: [w1708] -> w1704
          tunnel: [w1709] -> w1702
          tunnel: [w1710] -> w1699
          tunnel: w1698 -> [w1710]
          tunnel: [w1713] -> w1705
          tunnel: w1704 -> [w1713]
          tunnel: [w1712] -> w1703
          tunnel: w1702 -> [w1712]
          tunnel: w1699 -> [w1711]
          tunnel: [w1722] -> w1701
          tunnel: w1705 -> [w1742]
          tunnel: w1703 -> [w1739]
          tunnel: [w1731] -> w1700
          frame #0 {
            n819 = call "Loop Timer8"("Count(Ticks)"=w1709) -> ("Tick Count(Ticks)"=w1708:u32)
          }
          frame #1 {
            # "Then to PRL 440 amp"
            n820 = xnode "FPGA I/O Node"("Connector1/DIO32"=w1711) -> ()  [unwired: 1 in, 1 out]
          }
          frame #2 {
            n821 = feedback-in #76(w1742) -> ()
            n822 = feedback #76(w1742) -> (w1741:u32)
            n823 = Subtract(x=w1742, y=w1741) -> (x-y=w1740:u32)
            n824 = Subtract(x=w1740, y=w1739) -> (x-y=w1715:u32)
            n825 = Number To Boolean Array(number=w1715) -> (Boolean array=w1716:bool[])
            n826 = Or Array Elements(Boolean array=w1716) -> (logical OR=w1714:bool)
            n827 = Boolean To (0,1)(Boolean="+ phase (RI)") -> (0, 1=w1727:i16)
            n828 = Multiply(x=w1727, y="Phase count adjustment (RI)") -> (x*y=w1724:i16)
            n829 = Boolean To (0,1)(Boolean=w1714) -> (0, 1=w1721:i16)
            n830 = To Unsigned Byte Integer(number=w1721) -> (unsigned 8bit integer=w1718:u8)
            n831 = feedback #77(i16 0) -> (w1725:i16)
            n832 = feedback #78(u8 0) -> (w1719:u8)
            n833 = Add(x=w1718, y=w1719) -> (x+y=w1717:u8)
            "RI Late Counter" <- w1717
            n834 = feedback-in #78(w1717) -> ()
            n835 = Subtract(x=w1725, y=w1724) -> (x-y=w1723:i16)
            "RI Relative phase" <- w1723
            n836 = feedback-in #77(w1723) -> ()
            n837 = feedback #79(TRUE) -> (w1734:bool)
            n838 = case shown="2" "Red Laser Operating Mode" {
              tunnel: [TRUE FALSE w1748] -> w1731
              tunnel: w1734 -> [_ _ w1745]
              frame 0, Default {
              }
              frame 1 {
              }
              frame 2 {
                n839 = Not(x=w1745) -> (.not. x?=w1747:bool)
                n840 = Select(t=w1747, s="Invert RI", f=w1745) -> (s? t:f=w1748:bool)
              }
            }
            n841 = Not(x=w1734) -> (.not. x?=w1730:bool)
            n842 = Select(t="Red interlace ON count", s=w1730, f="Red interlace OFF count") -> (s? t:f=w1736:u16)
            n843 = Subtract(x=w1736, y=w1715) -> (x-y=w1728:u32)
            n844 = Add(x=w1728, y=w1724) -> (x+y=w1722:u32)
            n845 = feedback-in #79(w1730) -> ()
          }
        }
      }
      n846 = while "473 nm blue  fluorescent laser interlacing (DO to blue laser digital control input)." {
        shift-right: [w1597] -> _
        shift-left: w1580 -> [w1600]
        shift-right: [w1596] -> _
        shift-left: w1579 -> [w1594]
        shift-right: [w1589] -> _
        shift-left: _ -> [w1588]
        shift-right: [w1581] -> _
        shift-left: u16 0 -> [w1584]
        stop <- FALSE stop-if-true
        n847 = flat-sequence {
          tunnel: w1600 -> [w1603]
          tunnel: [w1602] -> w1599
          tunnel: [w1603] -> w1598
          tunnel: [w1606] -> w1595
          tunnel: w1594 -> [w1606]
          tunnel: w1588 -> [w1605]
          tunnel: [w1605] -> w1587
          tunnel: [w1604] -> w1585
          tunnel: w1584 -> [w1604]
          tunnel: [w1611] -> w1593
          tunnel: w1599 -> [w1611]
          tunnel: [w1610] -> w1592
          tunnel: w1598 -> [w1610]
          tunnel: w1595 -> [w1609]
          tunnel: w1587 -> [w1608]
          tunnel: [w1608] -> w1586
          tunnel: w1585 -> [w1607]
          tunnel: [w1607] -> w1583
          tunnel: [w1616] -> w1591
          tunnel: [w1615] -> w1590
          tunnel: w1592 -> [w1615]
          tunnel: w1593 -> [w1616]
          tunnel: w1586 -> [w1614]
          tunnel: w1583 -> [w1613]
          tunnel: [w1612] -> w1582
          tunnel: [w1673] -> w1597
          tunnel: w1591 -> [w1691]
          tunnel: w1590 -> [w1688]
          tunnel: [w1661] -> w1596
          tunnel: [w1659] -> w1589
          tunnel: w1582 -> [w1656]
          tunnel: [w1657] -> w1581
          frame #0 {
            n848 = call "Loop Timer7"("Count(Ticks)"=w1603) -> ("Tick Count(Ticks)"=w1602:u32)
          }
          frame #1 {
            n849 = xnode "FPGA I/O Node"("Connector1/DIO28"=w1609) -> ()  [unwired: 1 in, 1 out]
          }
          frame #2 {
            n850 = case shown="True" w1614 {
              tunnel: w1613 -> [w1617 w1619]
              tunnel: [w1617 w1618] -> w1612
              frame False {
              }
              frame True {
                n851 = flat-sequence {
                  tunnel: [w1625] -> w1622
                  tunnel: [w1624] -> w1621
                  tunnel: [w1623] -> w1620
                  tunnel: w1619 -> [w1623]
                  tunnel: w1622 -> [w1642]
                  tunnel: w1621 -> [w1639]
                  tunnel: w1620 -> [w1641]
                  tunnel: [w1640] -> w1618
                  frame #0 {
                    # "5 ns timing resolution"
                    n852 = node-c288() -> (w1628:T7)  [unwired: 1 in]
                    n853 = timed-loop {
                      timing: w1628 -> [_]
                      timing-out: [_] -> w1627
                      tunnel: "Lifetime timeout APD1" -> [w1634]
                      tunnel: [w1629] -> w1624
                      tunnel: [w1630] -> w1625
                      i -> [w1631]
                      stop <- w1633 stop-if-true
                      n854 = xnode "FPGA I/O Node"() -> ("Connector0/DIO5"=w1632:bool)  [unwired: 1 in, 1 out]
                      n855 = To Unsigned Word Integer(number=w1631) -> (unsigned 16bit integer=w1629:u16)
                      n856 = Equal?(x=w1634, y=w1629) -> (x = y?=w1630:bool)
                      n857 = Or(x=w1632, y=w1630) -> (x .or. y?=w1633:bool)
                    }
                    n858 = node-c288(w1627) -> ()
                  }
                  frame #1 {
                    n859 = Not(x=w1642) -> (.not. x?=w1643:bool)
                    n860 = case shown="True" w1643 {
                      tunnel: w1639 -> [_ w1645]
                      tunnel: w1641 -> [w1644 w1647]
                      tunnel: [w1644 w1646] -> w1640
                      frame False {
                        # "timed out, do nothing"
                      }
                      frame True {
                        # "photon detected,record time"
                        n861 = case shown="True" "Lifetime to FIFO" {
                          tunnel: w1645 -> [_ w1653]
                          tunnel: w1647 -> [w1649 w1651]
                          tunnel: [w1649 w1650] -> w1646
                          frame False {
                            # "don't record time\n(can't if doing force feedback)"
                          }
                          frame True {
                            # "number of events in fifo"
                            n862 = xnode ("FIFO Method Node")("Element"=w1653, "Timeout"=0) -> ()  [unwired: 1 in, 2 out]
                            n863 = Increment(x=w1651) -> (x+1=w1650:u16)
                          }
                        }
                        "lifetime (ticks)" <- w1645
                      }
                    }
                  }
                }
              }
            }
          }
          frame #3 {
            # "Reading fifo is tricky here since\nunknown # of events"
            # "For lifetime measurement:\nInterlacing and pulse falling"
            n864 = feedback-in #80(w1691) -> ()
            n865 = feedback #80(w1691) -> (w1690:u32)
            n866 = Subtract(x=w1691, y=w1690) -> (x-y=w1689:u32)
            n867 = Subtract(x=w1689, y=w1688) -> (x-y=w1666:u32)
            n868 = Number To Boolean Array(number=w1666) -> (Boolean array=w1667:bool[])
            n869 = Or Array Elements(Boolean array=w1667) -> (logical OR=w1665:bool)
            n870 = Boolean To (0,1)(Boolean="+ phase (BI D)") -> (0, 1=w1678:i16)
            n871 = Multiply(x=w1678, y="Phase count adjustment (BI D)") -> (x*y=w1675:i16)
            n872 = Boolean To (0,1)(Boolean=w1665) -> (0, 1=w1672:i16)
            n873 = To Unsigned Byte Integer(number=w1672) -> (unsigned 8bit integer=w1669:u8)
            n874 = feedback #81(i16 0) -> (w1676:i16)
            n875 = feedback #82(u8 0) -> (w1670:u8)
            n876 = Add(x=w1669, y=w1670) -> (x+y=w1668:u8)
            "Blue Late Counter (D)" <- w1668
            n877 = feedback-in #82(w1668) -> ()
            n878 = Subtract(x=w1676, y=w1675) -> (x-y=w1674:i16)
            "BI Relative phase (D)" <- w1674
            n879 = feedback-in #81(w1674) -> ()
            n880 = feedback #83(TRUE) -> (w1683:bool)
            n881 = case shown="2" "Blue Laser Operating Mode (D)" {
              tunnel: [TRUE FALSE w1697] -> w1661
              tunnel: w1683 -> [_ _ w1694]
              frame 0, Default {
              }
              frame 1 {
              }
              frame 2 {
                n882 = Not(x=w1694) -> (.not. x?=w1696:bool)
                n883 = Select(t=w1696, s="Invert BI (D)", f=w1694) -> (s? t:f=w1697:bool)
              }
            }
            n884 = Subtract(x=w1656, y="Lifetime events to read blue") -> (x-y=w1654:u16)
            n885 = Not(x=w1683) -> (.not. x?=w1681:bool)
            n886 = Select(t="Blue interlace ON count (D)", s=w1681, f="Blue interlace OFF count (D)") -> (s? t:f=w1685:u16)
            n887 = Subtract(x=w1685, y=w1666) -> (x-y=w1679:u32)
            n888 = Add(x=w1679, y=w1675) -> (x+y=w1673:u32)
            n889 = feedback-in #83(w1681) -> ()
            n890 = Select(t=w1654, s="Lifetime read blue fifo", f=w1656) -> (s? t:f=w1657:u16)
            "lifetime events in fifo" <- w1657
            n891 = Equal?(x="Blue Laser Operating Mode (D)", y=u8 2) -> (x = y?=w1662:bool)
            n892 = Not(x=w1661) -> (.not. x?=w1660:bool)
            n893 = And(x=w1660, y=w1662) -> (x .and. y?=w1659:bool)
          }
        }
      }
    }
    frame Enabled {
    }
  }
